vi "Text control 2 v6.5_pump-specific.vi"() -> ()   [LabVIEW 2016]
panel:
  in  "Tab Control":enum32{"Main", "Other parameters"}(tab)
  out "Line running":i32
  out "Total lines":i32
  out "Path":path=path "C:/users/rlp38/09Apr2009LTtesting/test2.txt"
  out "I vs Vg":cluster{"Y data in":dbl[], "X data in":dbl[]}[](graph)
  out "Is max":dbl format="%.2e"
  out "Id max":dbl format="%.2e"
  out "Ig max":dbl format="%.2e"
  out "Imax vs time":cluster{"Y data in":dbl[], "X data in":dbl[]}[](graph)
  out "Imin vs time":cluster{"Y data in":dbl[], "X data in":dbl[]}[](graph)
  out "I vs Vd":cluster{"Y data in":dbl[], "X data in":dbl[]}[](graph)
  in  "Script":string="#-------------------------------------------------------\n# SPM pump cleaning script\n#\n# Version: 0.5\n# Author: Dimitrios Simatos\n# Last updated: 2018-01-05\n#-------------------------------------------------------\n# Description\n#\n# This script is designed to run the cleaning sequence of the SPM OEM pump.\n# This script needs to be run 4 times!\n#-------------------------------------------------------\n# Changes\n#\n# Placed initialization and hard stop commands in the beginning.\n#-------------------------------------------------------\n# Important points\n#\n# Never leave any liquid in the pump to dry after the experiments. If they dry, the residue may block the valve.\n# Always run the cleaning cycle after the experiments.\n# Use clockwise rotation when going up in valve port numbers and vice versa.\n#-------------------------------------------------------\n# Things to do before running the script\n#\n# Set time units to minutes.\n# Set filenames.\n# Replace the tubing, if necessary.\n#-------------------------------------------------------\n# Port connections\n#\n# Port 1: Waste\n# Port 2: Waste\n# Port 3: Various cleaning liquids\n# Port 4: Waste\n# Port 5: Waste\n# Port 6: Waste\n#\n# Between each of the 4 runs, the settings of Port 3 will change, according to the cleaning protocol.\n# The settings for Port 3 are:\n# 1st run: 1% v/v solution of sodium hypochlorite in ultrapure water\n# 2nd run: 0.1% w/v solution of sodium dodecyl sulfate in ultrapure water\n# 3rd run: Ultrapure water\n# 4th run: Waste (in air, not immersed in liquid)\n#-------------------------------------------------------\n# Cleaning protocol for the SPM OEM pump (from the manual)\n#\n# A cleaning procedure should be performed at the end of each day or in between two different experiments.\n# An effective cleaning can be performed in the following manner:\n# • Bleach solution to kill microorganisms\n# 1. Prepare a solution of 1% chlorine bleach and deionized water\n#    NOTE: Prepare a 1% v/v solution of sodium hypochlorite in deionized water\n# 2. Prepare a reservoir and place 1 tubing in the bleach solution and 5 tubings in a waste recipient\n# 3. Pick up the bleach solution through 1 port to entirely fill the syringe\n# 4. Sequentially output the syringe content through the remaining ports and throw it to the waste\n# 5. Repeat operation at least 2 times\n# • Detergent solution to remove debris\n# 1. Prepare a solution of 0.1% detergent and deionized water\n#    NOTE: Prepare a 0.1% w/v solution of sodium dodecyl sulfate in deionized water\n# 2. Move the tubing from the bleach solution reservoir and place it into a reservoir of detergent solution\n# 3. Pick up the detergent solution through 1 port to entirely fill the syringe\n# 4. Sequentially output the detergent solution through the remaining ports into the waste recipient\n# 5. Repeat operation at least 2 times\n# • Rinsing water to prepare the pump for your next experiment\n# 1. Move the tubing from the detergent solution reservoir and place it into a reservoir of deionized water\n# 2. Pick up the rinsing solution through 1 port to entirely fill the syringe\n# 3. Sequentially output the rinse water through the remaining ports into the waste recipient\n# 4. Repeat operation at least 2 times\n# • Replace the tubing, if necessary\n#-------------------------------------------------------\n# Pumping cycles and execution time\n#\n# Execution time for a single cycle: 6 x (1 min + 10 sec) = 7 minutes\n# Total execution time: 4 x 7 = 28 minutes\n# Since the script has to run 4 times, the cleaning lasts for: 4 x 28 = 112 minutes\n# Air must be the last to be pumped through the valve, to remove all liquids.\n# There are 4 pumping cycles. Each one draws a different liquid through port 3 and pumps it sequentially through ports 1,2,4,5,6.\n# During the sequential pumping, each port receives 200 ml of liquid (20% of the total syringe volume = 600 \"plunger units\")\n# The device must be disconnected from the port during the cleaning procedure.\n# All cycles are similar, except cycle 1 has the initialization command uncommented and the first report valve command commented.\n#-------------------------------------------------------\n# Volume of liquid needed\n#\n# Volume of liquid needed per cycle: 1 ml\n# Total volume of liquid needed per script run: 4 x 1 = 4 ml\n# Since the script has to run 4 times, the first 3 with different liquids, I need:\n# 4 ml of 1% v/v solution of sodium hypochlorite in ultrapure water\n# 4 ml of 0.1% w/v solution of sodium dodecyl sulfate in ultrapure water\n# 4 ml of ultrapure water\n#-------------------------------------------------------\n# Parameters\n#\n# Syringe size: 1 ml\n# Step resolution N = 0.01 mm\n# Drawing flow V = 300 pulses/second (6000 ul/min)\n# Pumping flow V = 300 pulses/second (6000 ul/min)\n#-------------------------------------------------------\n# Pump initialization\npump /1T #hard stop pump\npump /1ZR #initialize pump\n#-------------------------------------------------------\n# Cycle 1\n# Fill the syringe\npump /1Q #query pump\npump /1? #report absolute plunger position\n#pump /1?6 #report valve position\nwait-min 1 #wait 1 minute\npump /1N0R #set step resolution: 0.01 mm\npump /1Q #query pump\npump /1? #report absolute plunger position (the plunger should be at 0)\npump /1?6 #report valve position\nwait 1000 #wait 1 second\npump /1V300R #choose speed: 300 steps/s (6000 ul/min)\npump /1Q #query pump\nwait 1000 #wait 1 second\npump /1I3R #go to port 3, clockwise rotation\npump /1Q #query pump\npump /1?6 #report valve position\nwait 1000 #wait 1 second\npump /1A3000R #go to absolute position 3000 (= draw 1 ml)\nwait 30000 #wait 30 seconds\npump /1Q #query pump\npump /1? #report absolute plunger position (the plunger should have finished moving)\n#pump /1?6 #report valve position\n# The sequential pumping begins\n# Port 1\npump /1O1R #switch to port 1, counterclockwise rotation\npump /1Q #query pump\npump /1?6 #report valve position\npump /1A2400R #go to absolute position 2400 (= pump 200 ul)\npump /1Q #query pump\npump /1? #report absolute plunger position (the plunger should be moving to 0)\nwait-min 1 #wait 1 minute\npump /1? #report absolute plunger position (the plunger should have finished moving)\n# Port 2\npump /1I2R #switch to port 2, clockwise rotation\npump /1Q #query pump\npump /1?6 #report valve position\npump /1A1800R #go to absolute position 1800 (= pump 200 ul)\npump /1Q #query pump\npump /1? #report absolute plunger position (the plunger should be moving to 0)\nwait-min 1 #wait 1 minute\npump /1? #report absolute plunger position (the plunger should have finished moving)\n# Port 4\npump /1I4R #switch to port 4, clockwise rotation\npump /1Q #query pump\npump /1?6 #report valve position\npump /1A1200R #go to absolute position 1200 (= pump 200 ul)\npump /1Q #query pump\npump /1? #report absolute plunger position (the plunger should be moving to 0)\nwait-min 1 #wait 1 minute\npump /1? #report absolute plunger position (the plunger should have finished moving)\n# Port 5\npump /1I5R #switch to port 5, clockwise rotation\npump /1Q #query pump\npump /1?6 #report valve position\npump /1A600R #go to absolute position 600 (= pump 200 ul)\npump /1Q #query pump\npump /1? #report absolute plunger position (the plunger should be moving to 0)\nwait-min 1 #wait 1 minute\npump /1? #report absolute plunger position (the plunger should have finished moving)\n# Port 6\npump /1I6R #switch to port 6, clockwise rotation\npump /1Q #query pump\npump /1?6 #report valve position\npump /1A0R #go to absolute position 0 (= pump 200 ul)\npump /1Q #query pump\npump /1? #report absolute plunger position (the plunger should be moving to 0)\nwait-min 1 #wait 1 minute\npump /1? #report absolute plunger position (the plunger should have finished moving)\n#-------------------------------------------------------\n# Cycle 2\n# Fill the syringe\n#pump /1ZR #initialize pump\npump /1Q #query pump\npump /1? #report absolute plunger position\npump /1?6 #report valve position\nwait-min 1 #wait 1 minute\npump /1N0R #set step resolution: 0.01 mm\npump /1Q #query pump\npump /1? #report absolute plunger position (the plunger should be at 0)\npump /1?6 #report valve position\nwait 1000 #wait 1 second\npump /1V300R #choose speed: 300 steps/s (6000 ul/min)\npump /1Q #query pump\nwait 1000 #wait 1 second\npump /1O3R #go to port 3, counterclockwise rotation\npump /1Q #query pump\npump /1?6 #report valve position\nwait 1000 #wait 1 second\npump /1A3000R #go to absolute position 3000 (= draw 1 ml)\nwait 30000 #wait 30 seconds\npump /1Q #query pump\npump /1? #report absolute plunger position (the plunger should have finished moving)\n#pump /1?6 #report valve position\n# The sequential pumping begins\n# Port 1\npump /1O1R #switch to port 1, counterclockwise rotation\npump /1Q #query pump\npump /1?6 #report valve position\npump /1A2400R #go to absolute position 2400 (= pump 200 ul)\npump /1Q #query pump\npump /1? #report absolute plunger position (the plunger should be moving to 0)\nwait-min 1 #wait 1 minute\npump /1? #report absolute plunger position (the plunger should have finished moving)\n# Port 2\npump /1I2R #switch to port 2, clockwise rotation\npump /1Q #query pump\npump /1?6 #report valve position\npump /1A1800R #go to absolute position 1800 (= pump 200 ul)\npump /1Q #query pump\npump /1? #report absolute plunger position (the plunger should be moving to 0)\nwait-min 1 #wait 1 minute\npump /1? #report absolute plunger position (the plunger should have finished moving)\n# Port 4\npump /1I4R #switch to port 4, clockwise rotation\npump /1Q #query pump\npump /1?6 #report valve position\npump /1A1200R #go to absolute position 1200 (= pump 200 ul)\npump /1Q #query pump\npump /1? #report absolute plunger position (the plunger should be moving to 0)\nwait-min 1 #wait 1 minute\npump /1? #report absolute plunger position (the plunger should have finished moving)\n# Port 5\npump /1I5R #switch to port 5, clockwise rotation\npump /1Q #query pump\npump /1?6 #report valve position\npump /1A600R #go to absolute position 600 (= pump 200 ul)\npump /1Q #query pump\npump /1? #report absolute plunger position (the plunger should be moving to 0)\nwait-min 1 #wait 1 minute\npump /1? #report absolute plunger position (the plunger should have finished moving)\n# Port 6\npump /1I6R #switch to port 6, clockwise rotation\npump /1Q #query pump\npump /1?6 #report valve position\npump /1A0R #go to absolute position 0 (= pump 200 ul)\npump /1Q #query pump\npump /1? #report absolute plunger position (the plunger should be moving to 0)\nwait-min 1 #wait 1 minute\npump /1? #report absolute plunger position (the plunger should have finished moving)\n#-------------------------------------------------------\n# Cycle 3\n# Fill the syringe\n#pump /1ZR #initialize pump\npump /1Q #query pump\npump /1? #report absolute plunger position\npump /1?6 #report valve position\nwait-min 1 #wait 1 minute\npump /1N0R #set step resolution: 0.01 mm\npump /1Q #query pump\npump /1? #report absolute plunger position (the plunger should be at 0)\npump /1?6 #report valve position\nwait 1000 #wait 1 second\npump /1V300R #choose speed: 300 steps/s (6000 ul/min)\npump /1Q #query pump\nwait 1000 #wait 1 second\npump /1O3R #go to port 3, counterclockwise rotation\npump /1Q #query pump\npump /1?6 #report valve position\nwait 1000 #wait 1 second\npump /1A3000R #go to absolute position 3000 (= draw 1 ml)\nwait 30000 #wait 30 seconds\npump /1Q #query pump\npump /1? #report absolute plunger position (the plunger should have finished moving)\n#pump /1?6 #report valve position\n# The sequential pumping begins\n# Port 1\npump /1O1R #switch to port 1, counterclockwise rotation\npump /1Q #query pump\npump /1?6 #report valve position\npump /1A2400R #go to absolute position 2400 (= pump 200 ul)\npump /1Q #query pump\npump /1? #report absolute plunger position (the plunger should be moving to 0)\nwait-min 1 #wait 1 minute\npump /1? #report absolute plunger position (the plunger should have finished moving)\n# Port 2\npump /1I2R #switch to port 2, clockwise rotation\npump /1Q #query pump\npump /1?6 #report valve position\npump /1A1800R #go to absolute position 1800 (= pump 200 ul)\npump /1Q #query pump\npump /1? #report absolute plunger position (the plunger should be moving to 0)\nwait-min 1 #wait 1 minute\npump /1? #report absolute plunger position (the plunger should have finished moving)\n# Port 4\npump /1I4R #switch to port 4, clockwise rotation\npump /1Q #query pump\npump /1?6 #report valve position\npump /1A1200R #go to absolute position 1200 (= pump 200 ul)\npump /1Q #query pump\npump /1? #report absolute plunger position (the plunger should be moving to 0)\nwait-min 1 #wait 1 minute\npump /1? #report absolute plunger position (the plunger should have finished moving)\n# Port 5\npump /1I5R #switch to port 5, clockwise rotation\npump /1Q #query pump\npump /1?6 #report valve position\npump /1A600R #go to absolute position 600 (= pump 200 ul)\npump /1Q #query pump\npump /1? #report absolute plunger position (the plunger should be moving to 0)\nwait-min 1 #wait 1 minute\npump /1? #report absolute plunger position (the plunger should have finished moving)\n# Port 6\npump /1I6R #switch to port 6, clockwise rotation\npump /1Q #query pump\npump /1?6 #report valve position\npump /1A0R #go to absolute position 0 (= pump 200 ul)\npump /1Q #query pump\npump /1? #report absolute plunger position (the plunger should be moving to 0)\nwait-min 1 #wait 1 minute\npump /1? #report absolute plunger position (the plunger should have finished moving)\n#-------------------------------------------------------\n# Cycle 4\n# Fill the syringe\n#pump /1ZR #initialize pump\npump /1Q #query pump\npump /1? #report absolute plunger position\npump /1?6 #report valve position\nwait-min 1 #wait 1 minute\npump /1N0R #set step resolution: 0.01 mm\npump /1Q #query pump\npump /1? #report absolute plunger position (the plunger should be at 0)\npump /1?6 #report valve position\nwait 1000 #wait 1 second\npump /1V300R #choose speed: 300 steps/s (6000 ul/min)\npump /1Q #query pump\nwait 1000 #wait 1 second\npump /1O3R #go to port 3, counterclockwise rotation\npump /1Q #query pump\npump /1?6 #report valve position\nwait 1000 #wait 1 second\npump /1A3000R #go to absolute position 3000 (= draw 1 ml)\nwait 30000 #wait 30 seconds\npump /1Q #query pump\npump /1? #report absolute plunger position (the plunger should have finished moving)\n#pump /1?6 #report valve position\n# The sequential pumping begins\n# Port 1\npump /1O1R #switch to port 1, counterclockwise rotation\npump /1Q #query pump\npump /1?6 #report valve position\npump /1A2400R #go to absolute position 2400 (= pump 200 ul)\npump /1Q #query pump\npump /1? #report absolute plunger position (the plunger should be moving to 0)\nwait-min 1 #wait 1 minute\npump /1? #report absolute plunger position (the plunger should have finished moving)\n# Port 2\npump /1I2R #switch to port 2, clockwise rotation\npump /1Q #query pump\npump /1?6 #report valve position\npump /1A1800R #go to absolute position 1800 (= pump 200 ul)\npump /1Q #query pump\npump /1? #report absolute plunger position (the plunger should be moving to 0)\nwait-min 1 #wait 1 minute\npump /1? #report absolute plunger position (the plunger should have finished moving)\n# Port 4\npump /1I4R #switch to port 4, clockwise rotation\npump /1Q #query pump\npump /1?6 #report valve position\npump /1A1200R #go to absolute position 1200 (= pump 200 ul)\npump /1Q #query pump\npump /1? #report absolute plunger position (the plunger should be moving to 0)\nwait-min 1 #wait 1 minute\npump /1? #report absolute plunger position (the plunger should have finished moving)\n# Port 5\npump /1I5R #switch to port 5, clockwise rotation\npump /1Q #query pump\npump /1?6 #report valve position\npump /1A600R #go to absolute position 600 (= pump 200 ul)\npump /1Q #query pump\npump /1? #report absolute plunger position (the plunger should be moving to 0)\nwait-min 1 #wait 1 minute\npump /1? #report absolute plunger position (the plunger should have finished moving)\n# Port 6\npump /1I6R #switch to port 6, clockwise rotation\npump /1Q #query pump\npump /1?6 #report valve position\npump /1A0R #go to absolute position 0 (= pump 200 ul)\npump /1Q #query pump\npump /1? #report absolute plunger position (the plunger should be moving to 0)\nwait-min 1 #wait 1 minute\npump /1? #report absolute plunger position (the plunger should have finished moving)\n#-------------------------------------------------------"
  out "Command running:":string
  out "Serial port data":string
  out "Elapsed Time":dbl caption="Elapsed Time (s)"
  in  "Time Units":u16(ring)=1 items=["Seconds", "Minutes", "Hours"]
  in  "Time Offset":dbl caption="Set Start Time (s)"
  in  "Reset":bool
  in  "Auto Reset":bool
  in  "integration time":u32(slide) max=2 step=1 scale=0.0..2.0
  in  "Interrupt scan":bool
  out "Absolute plunger position vs time":cluster{"Y data in":dbl[], "X data in":dbl[]}[](graph)
  out "Valve position vs time":cluster{"Y data in":dbl[], "X data in":dbl[]}[](graph)
  out "Is on":dbl format="%.2e"
  out "Id on":dbl format="%.2e"
  out "Ig on":dbl format="%.2e"
  out "Ion vs time":cluster{"Y data in":dbl[], "X data in":dbl[]}[](graph)
  out "Ioff vs time":cluster{"Y data in":dbl[], "X data in":dbl[]}[](graph)
  out "Ig min":dbl format="%.2e"
  out "Id min":dbl format="%.2e"
  out "Is min":dbl format="%.2e"
  out "Is off":dbl format="%.2e"
  out "Id off":dbl format="%.2e"
  out "Ig off":dbl format="%.2e"
  in  "Integration time (long)":dbl=0.32 min=0.04 max=2.0 step=0.02 format="%.2f"
  in  "Integration time (short)":dbl=0.0019 min=8e-05 max=0.0019 step=8e-05 format="%^.0e"
  in  "Gate: Compliance":dbl=0.001 format="%.8f"
  in  "Drain: Compliance":dbl=0.001 format="%.8f"
  in  "Hard stop pump":bool
  in  "Halt pump":bool
  in  "Interrupt program":bool
  in  "Suffix (script)":string="step_1_up-H2O_initial_script.txt"
  in  "Filename (variable part)":string="step_1_up-H2O_initial_"
  in  "Plot output curve extrema vs time":bool
  in  "Plot transfer curve extrema vs time":bool=TRUE
  in  "Gate Range\nmode":u16(ring) items=["Auto", "Limited", "Fixed"]
  in  "Gate Range":u8(slide)=6 max=11 scale=0.0..11.0
  in  "Source/Drain\nRange mode":u16(ring) items=["Auto", "Limited", "Fixed"]
  in  "Source/Drain Range":u8(slide)=6 max=11 scale=0.0..11.0
  in  "Panel Controls":T1={"Emergency Stop"=refnum, "TransGraph Max"=1e-05, "Text/Graph (text=false)"=TRUE} {"TransGraph Max" format="%.2e"}
  in  "Panel Controls 2":T2={"Emergency Stop"=refnum, "TransGraph Max"=1e-05, "Text/Graph (text=false)"=TRUE, "TransGraph Min"=1e-11} {"TransGraph Min" format="%.2e"; "TransGraph Max" format="%.2e"}
  in  "SMU4":cluster{"on/off":bool, "Voltage":dbl} {"Voltage" min=-100.0 max=100.0 format="%.2f"}
  in  "Full Reset":bool
  in  "Standby":T3
  out "error out":errorcluster
  in  "Delay before read (ms)":u32=1000
  in  "byte count":u32=64
  in  "Serial End Mode for Reads":u16(ring)=2 items=["None", "LastBit", "TermChar"]
  in  "Timeout (ms)":u32=10000
  in  "Enable Termination\nChar (T)":bool=TRUE
  in  "Termination char\n(0xA = '\\n' = LF)\n(0xD = '\\r' = CR)":u8=13 format="%.0x"
  in  "flow control":u16(ring) items=["None"=0, "XON/XOFF"=1, "RTS/CTS"=2, "DTR/DSR"=4]
  in  "stop bits":u16(ring)=10 items=["1.0"=10, "1.5"=15, "2.0"=20]
  in  "parity":u16(ring) items=["None", "Odd", "Even", "Mark", "Space"]
  in  "data bits":u16=8 min=5 max=8 step=1
  in  "VISA resource name":refnum<visa-resource-name>="COM6"
  in  "baud rate":u32=9600
  out "Timings Indicator":T4
  in  "Timings (overwritten by the Front Panel)":T5={"integration time"=0, "Short/Long integration time"=0.00064, "hold time (sec)"=0.0, "delay time (sec)"=0.0, "Step Time (0 disables)"=0.0, "sweep method"=0, "Pulse period"=0.005, "Base voltage"=0.0, "Pulse width"=0.0005} {"Pulse width" min=0.0005 max=0.1 step=0.0001 format="%.4f"; "Base voltage" format="%^.4e"; "Pulse period" min=0.005 max=1.0 step=0.0001 format="%.4f"; "sweep method" items=["Continuous", "Pulsed"]; "Step Time (0 disables)" format="%.2f"; "delay time (sec)" format="%.4f"; "hold time (sec)" format="%.4f"; "Short/Long integration time" format="%^.0e"; "integration time" scale=0.0..2.0}
  out "SMU4 Indicator":cluster{"on/off":bool, "Voltage":dbl} {"Voltage" min=-100.0 max=100.0 format="%.2f"}
  in  "Gate":T6={"Gate Start"=0.0, "Gate Stop"=2.0, "Gate Step (linear only)"=1.0, "Gate Compliance"=0.0001, "Gate PComp"=0.0, "Range mode"=0, "Range"=6} {"Range" max=11 scale=0.0..11.0; "Range mode" items=["Auto", "Limited", "Fixed"]; "Gate PComp" format="%^.2e"; "Gate Compliance" format="%^.2e"; "Gate Step (linear only)" format="%^.4e"; "Gate Stop" format="%^.4e"; "Gate Start" format="%^.4e"}
  in  "Drain 2":T7={"Drain Start"=0.0, "Drain Stop"=2.0, "Drain Compliance"=0.0001, "Drain Step"=1.0, "Drain PComp"=0.0, "Range mode"=0, "Range"=6} {"Range" max=11 scale=0.0..11.0; "Range mode" items=["Auto", "Limited", "Fixed"]; "Drain PComp" format="%^.2e"; "Drain Step" format="%^.4e"; "Drain Compliance" format="%^.2e"; "Drain Stop" format="%^.4e"; "Drain Start" format="%^.4e"}
  # "Syntax:\nitime [s|m|l] time(sec): [s|m|l] determines the integration time setting (small|medium|long) and time sets the value.\nNOTE: The value of the integration time has to be within the range allowed by its category (s|m|l), otherwise, the closest value will be used. (e.g. if the category is set to short but the time value is very long, the actual value used will be the maximum short integration time.\nIntegration times:\n    Short: Default: 640 us. Range: 8E-5 - 1.92E-3 seconds.\n    Medium: Fixed at 1 NPL cycle (0.02 seconds).\n    Long: Default: 16 NPL cycles (0.32 seconds). Range: 2-100 NPL cycles (0.04 seconds - 2 seconds).\ngaterangemode [a|l|f]\ndrainrangemode [a|l|f]\npulsed [on|off] PulsePeriod(sec) PulseBaseVoltage PulseONWidth(sec)\nstandby [on l off]\nwait NumMilliseconds\nwait-min NumMinutes\n# texthere = comment\nSMU4 [ON|OFF] Voltage\ntransfer [s|d] VgStart VgStop VgStep VdStart VdStop VdStep\noutput [s|d] VgStart VgStop VgStep VdStart VdStop VdStep\nsample Vg Vd NumSamples Time(s) SampleInterval(s)\nsamplei Idg NumSamples Time(s) SampleInterval(s) VDGcompliance\n100 samples is approximately 13 seconds with medium integration\n# if in doubt use SampleInterval(s) = 0.004\nstressV VG VD IGcompliance IDcompliance Duration(sec)\nstressI IDG VDGcompliance Duration(sec)\nvsu2pulse Bias Duration(s)\npulsedstressV [s|d] VEstop VgON VgOFF Period(s) PulseONwidth(s) Vd\nsample-fpp Vg Vd NumSamples Time\nresample-fpp Vg Vd\ntransfer-fpp [s|d] VgStart VgStop VgStep VdStart VdStop VdStep\noutput-fpp [s|d] VgStart VgStop VgStep VdStart VdStop VdStep\nserial SerialPortCommand\npump SerialPortCommand for the SPM pump\n\nSPM Pump Syntax (<x>: pump number, use 1 if only one pump):\nif the command syntax contains [R], then append the letter R to the command\n/<x>Q: query (a query command should follow each command)\n/<x>Z[R] or /<x>Y[R]: initialize pump\n/<x>N<n>[R] (<n>=0,1): <0> (<1>) microstep 0.01 mm (0.00125 mm) resolution\n/<x>I<n> (<n>=0-6): turn to port number n (clockwise)\n/<x>O<n> (<n>=0-6): turn to port number n (counterclockwise)\n/<x>X: Re-execute last command string\n/<x>G<n>[R] (<n>=0-60000): repeat command sequence (default: 0, 0=loop forever)\n/<x>g: Mark the start of a repeat sequence (max = 10)\n/<x>M<n>[R] (<n>=0-86400000): delay command execution by n milliseconds\n/<x>H: Halt; Pause the sequence after finishing the current move\n/<x>T: Hardstop; Interrupt the current move and suppress it from the sequence\n/<x>A<n>[R] (<n>=0-3000 with N=0, 0-24000 with N=1): absolute position\n/<x>P<n>[R] (<n>=0-3000 with N=0, 0-24000 with N=1): relative pickup\n/<x>D<n>[R] (<n>=0-3000 with N=0, 0-24000 with N=1): relative dispense\n/<x>V<n>[R] (<n>=1-1600 default: 150): set peak speed (pulses/sec)\nNOTE: The lowest speed limit is 1 pulse/sec, not 5, as the manual states.\n/<x>S<n>[R] (<n>=10-40 default: 22): set speed (NOT in pulses/sec, look in manual)\nNOTE: When controlled with absolute position, one does not need to pay special attention to the syringe that is mounted on the pump.\nWithdraw from lower stage (ports 3, 5), dispense from higher stage (ports 2, 4, 6).\nConnect Port 1 to waste."
  # "Time"
  # "1\n2\n3\n4\n5\n6\n7\n8\n9\n10\n11\n12\n13\n14\n15\n16\n17\n18\n19\n20"
  # "Serial port settings"
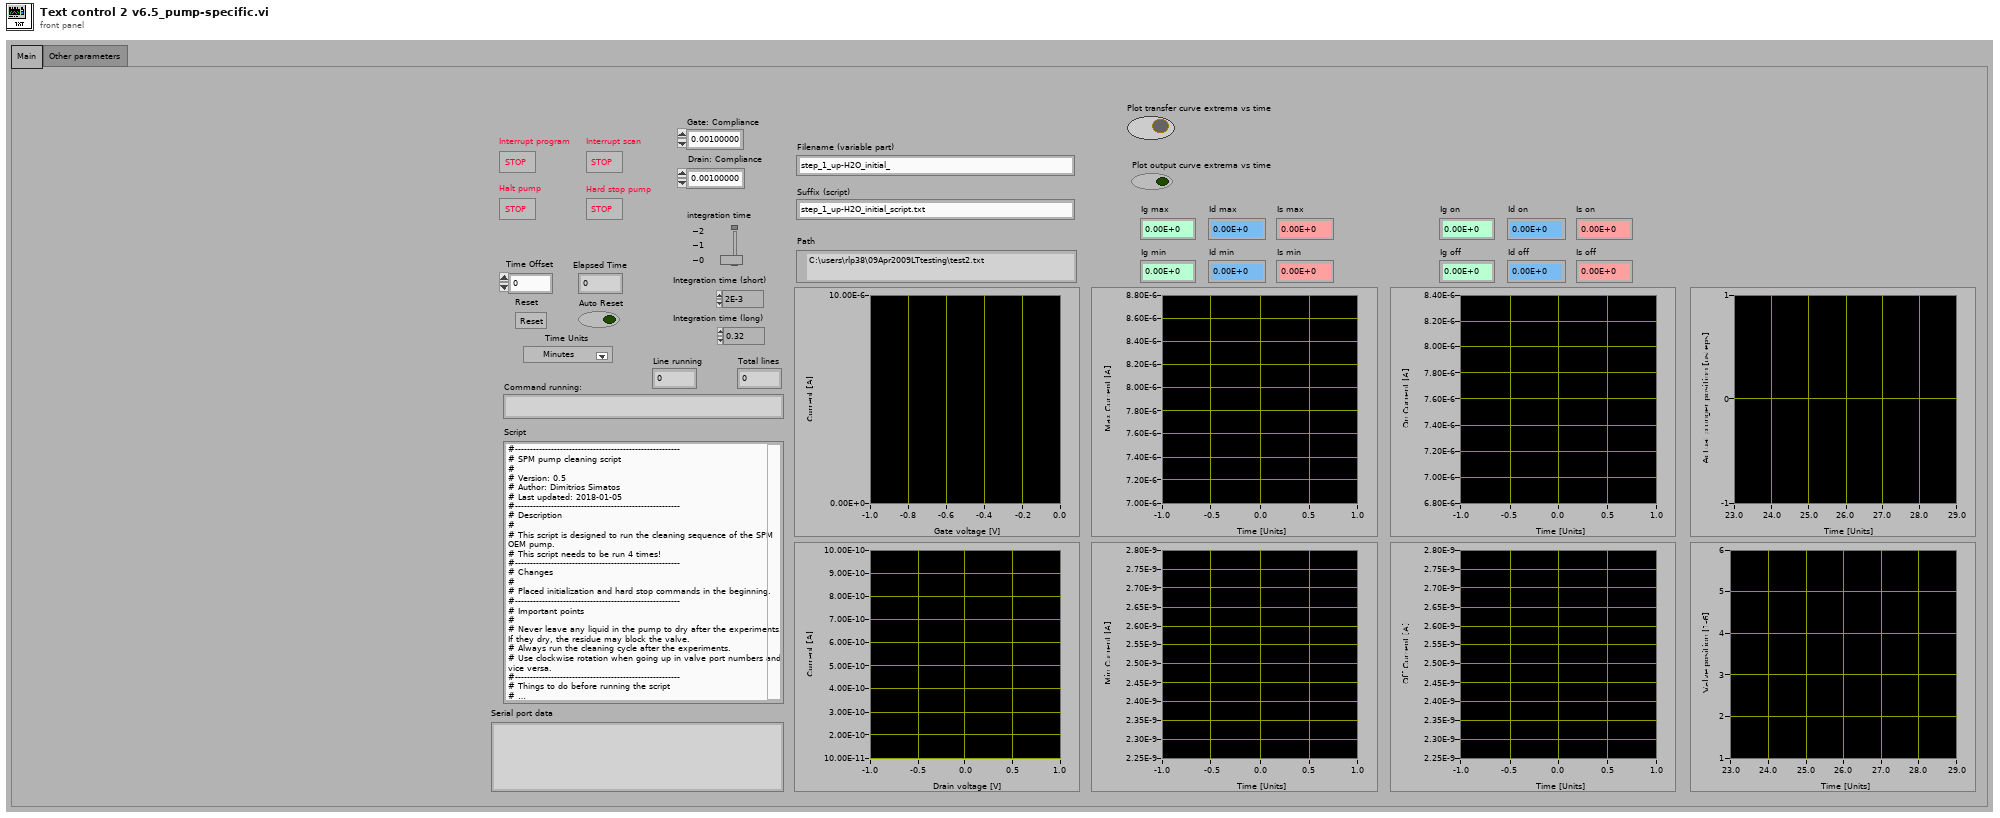
[diagram p1: front panel]
types:
  T1 = cluster{"Emergency Stop":refnum<vi>, "TransGraph Max":dbl, "Text/Graph (text=false)":bool}
  T2 = cluster{"Emergency Stop":refnum<vi>, "TransGraph Max":dbl, "Text/Graph (text=false)":bool, "TransGraph Min":dbl}
  T3 = cluster{"Gate Standby":bool, "Drain Standby":bool}
  T4 = cluster{"integration time (0:s, 1:m, 2:l)":u32, "Short/Long integration time":dbl, "hold time (sec)":dbl, "delay time (sec)":dbl, "Step Time (0 disables)":dbl, "sweep method":u16, "Pulse period":dbl, "Base voltage":dbl, "Pulse width":dbl}
  T5 = cluster{"integration time":u32, "Short/Long integration time":dbl, "hold time (sec)":dbl, "delay time (sec)":dbl, "Step Time (0 disables)":dbl, "sweep method":u16, "Pulse period":dbl, "Base voltage":dbl, "Pulse width":dbl}
  T6 = cluster{"Gate Start":dbl, "Gate Stop":dbl, "Gate Step (linear only)":dbl, "Gate Compliance":dbl, "Gate PComp":dbl, "Range mode":u16, "Range":u8}
  T7 = cluster{"Drain Start":dbl, "Drain Stop":dbl, "Drain Compliance":dbl, "Drain Step":dbl, "Drain PComp":dbl, "Range mode":u16, "Range":u8}
  T8 = enum16{"open", "replace", "create", "open or create", "replace or create", "replace or create with confirmation"}
  T9 = cluster{"V2 Start":dbl, "V2 Step":dbl, "Number of points":i32}
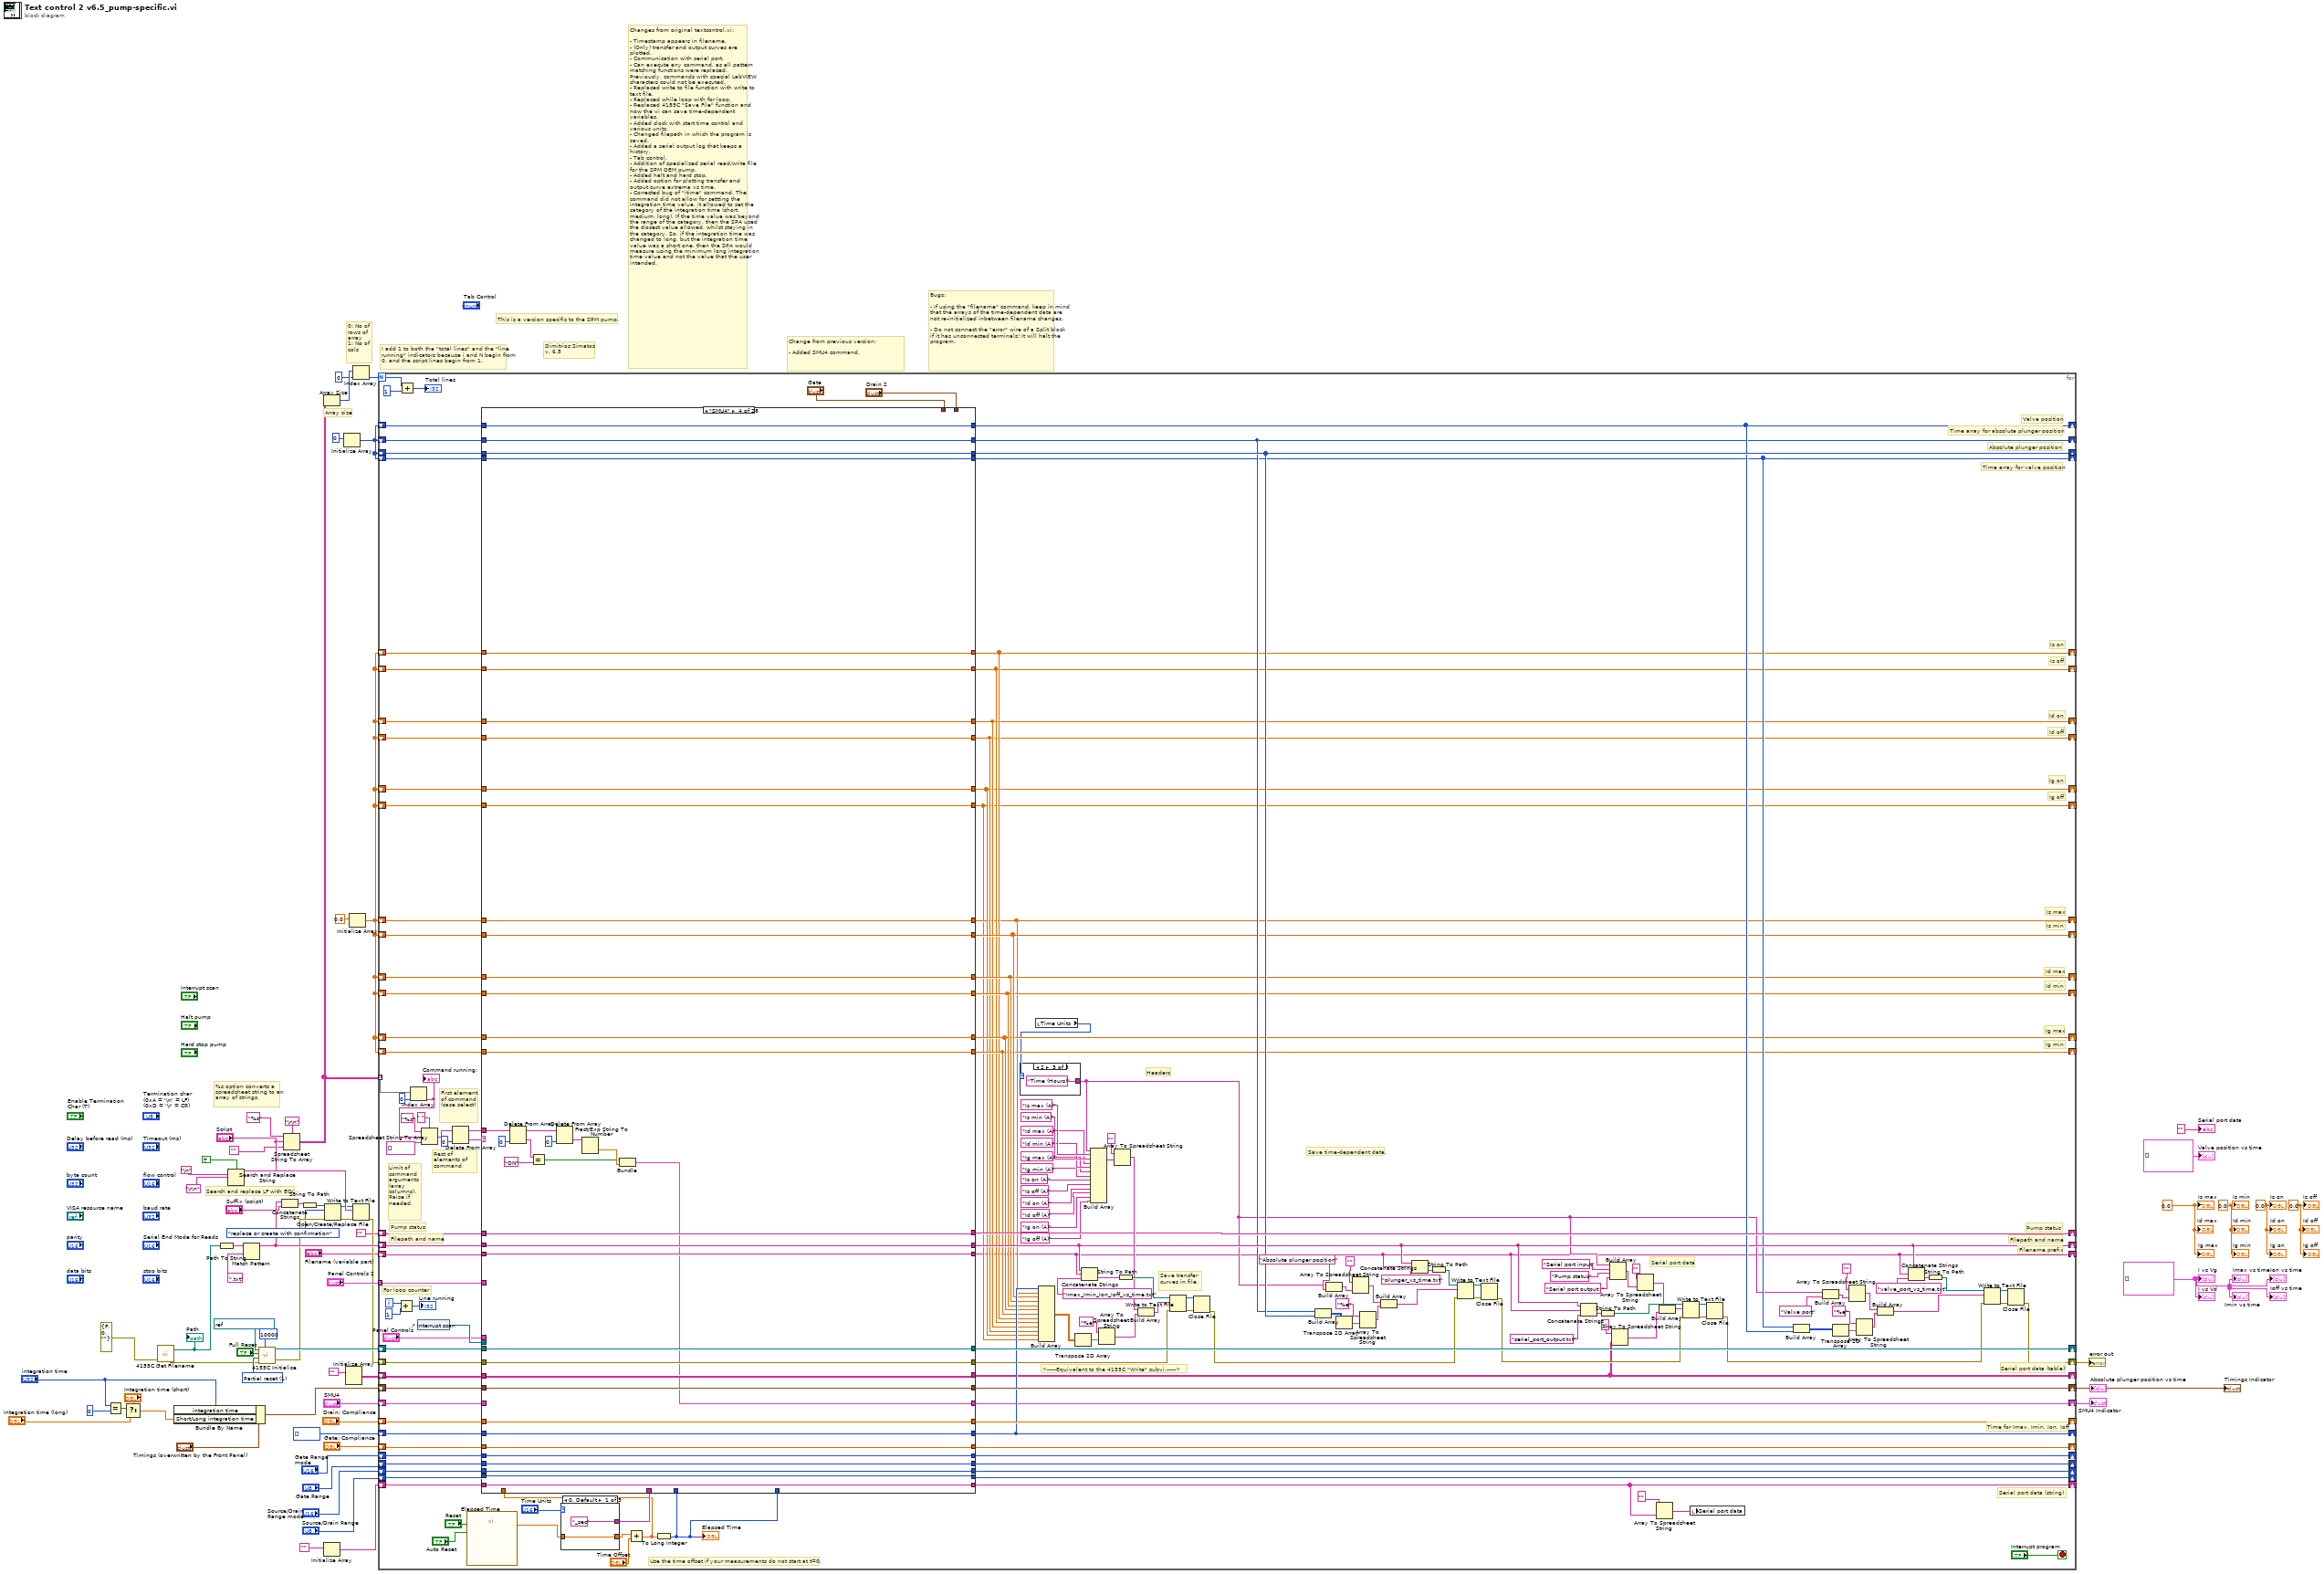
[diagram p0: block diagram]
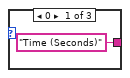
[diagram p2: hidden frame]
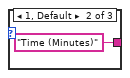
[diagram p3: hidden frame]
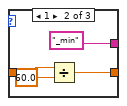
[diagram p4: hidden frame]
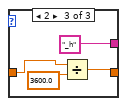
[diagram p5: hidden frame]
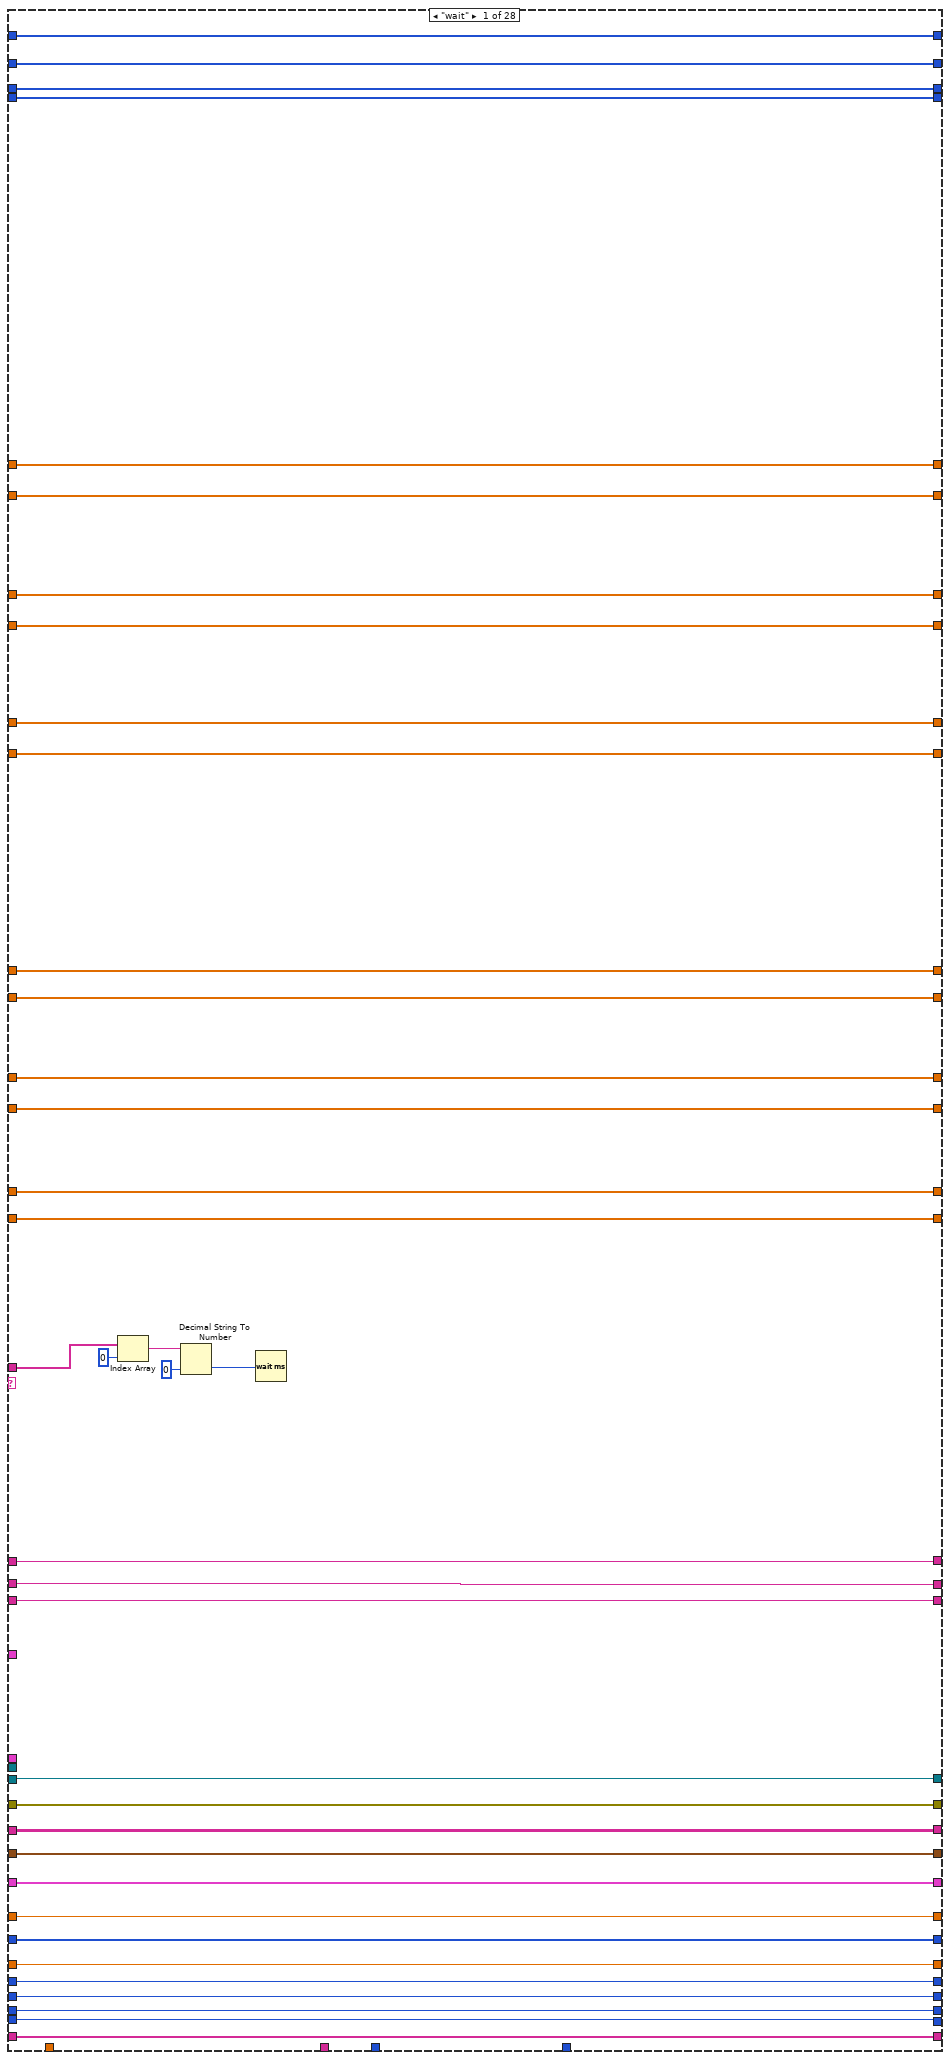
[diagram p6: hidden frame]
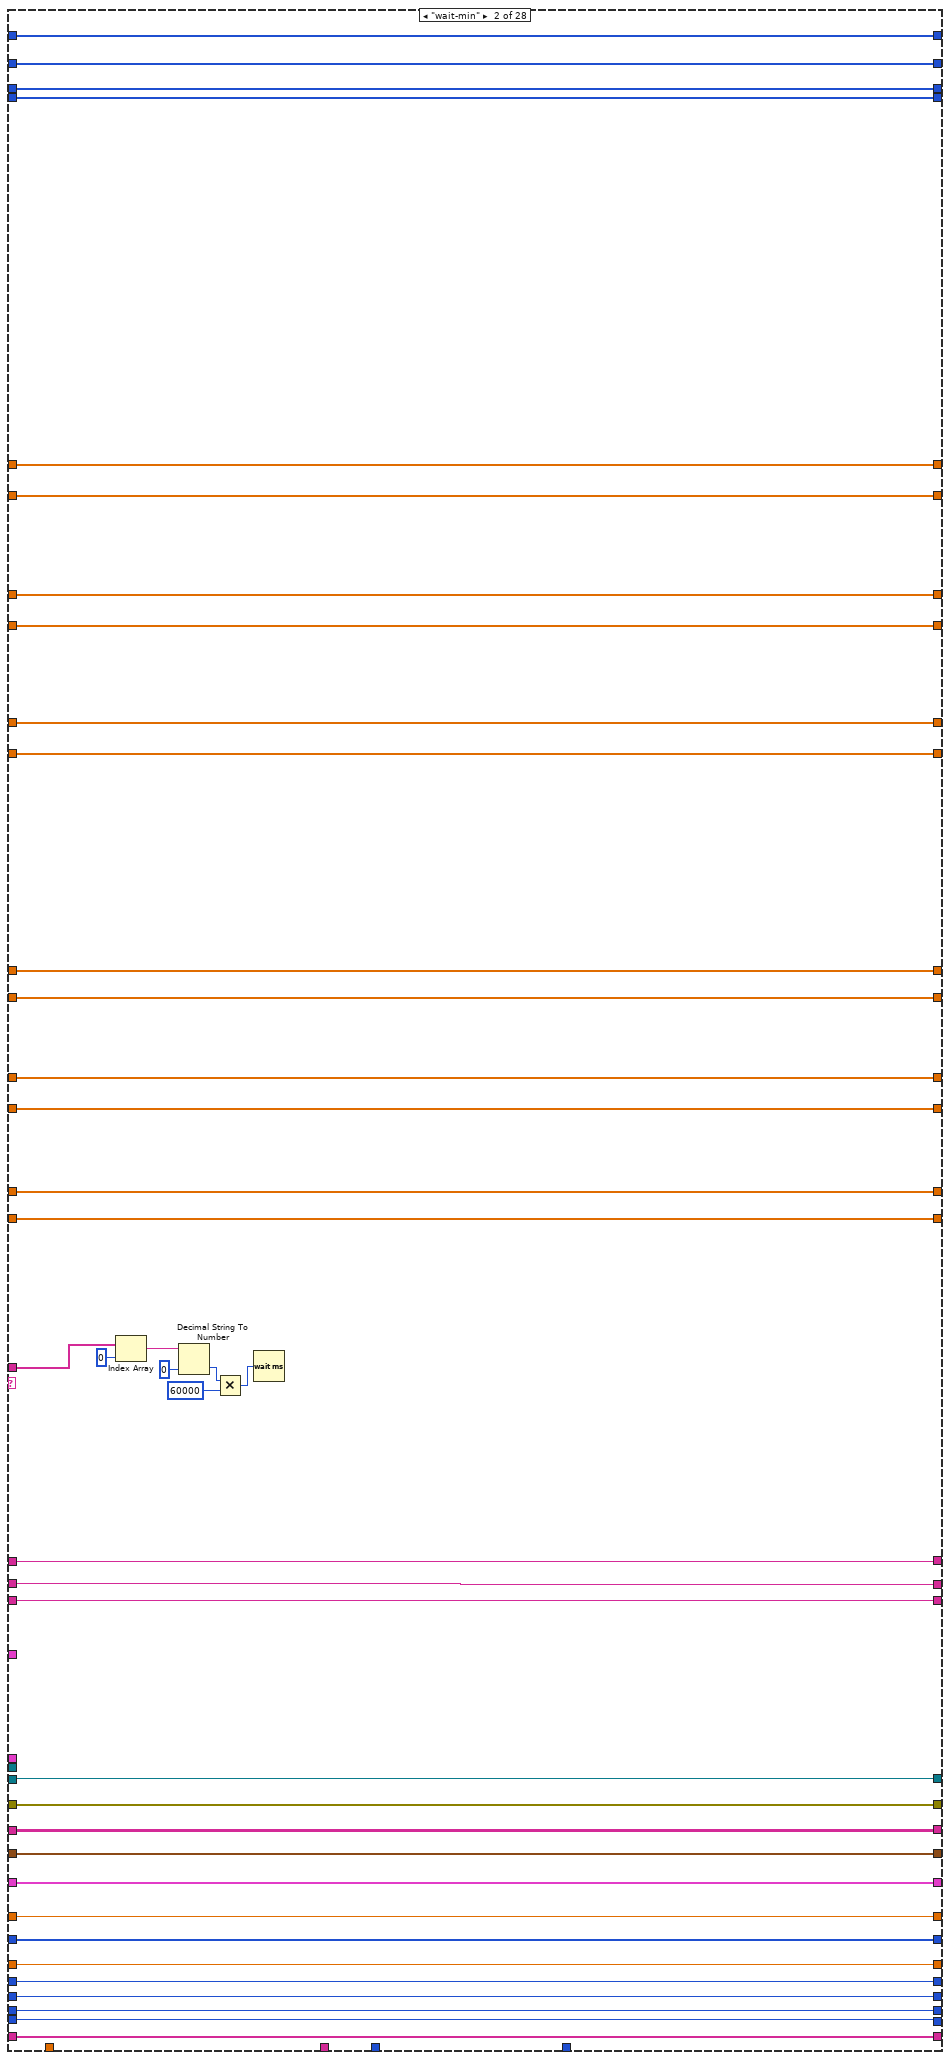
[diagram p7: hidden frame]
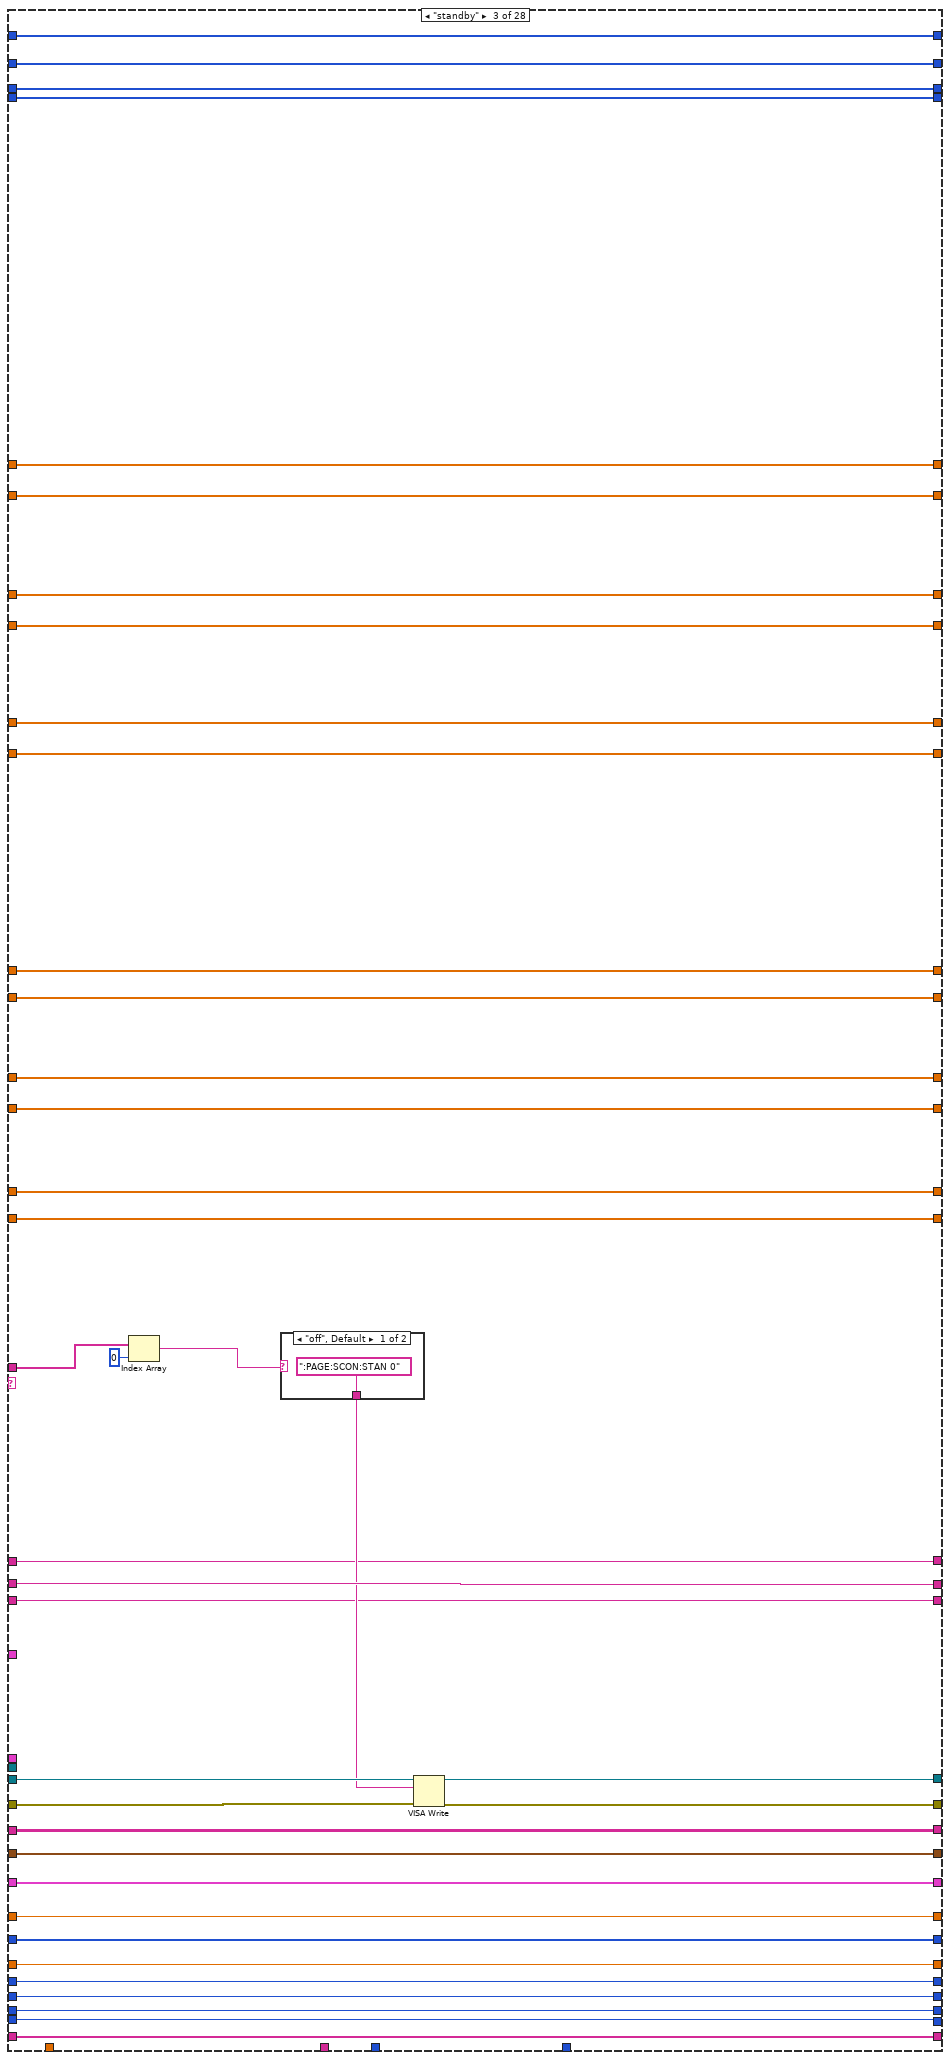
[diagram p8: hidden frame]
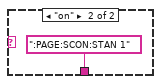
[diagram p9: hidden frame]
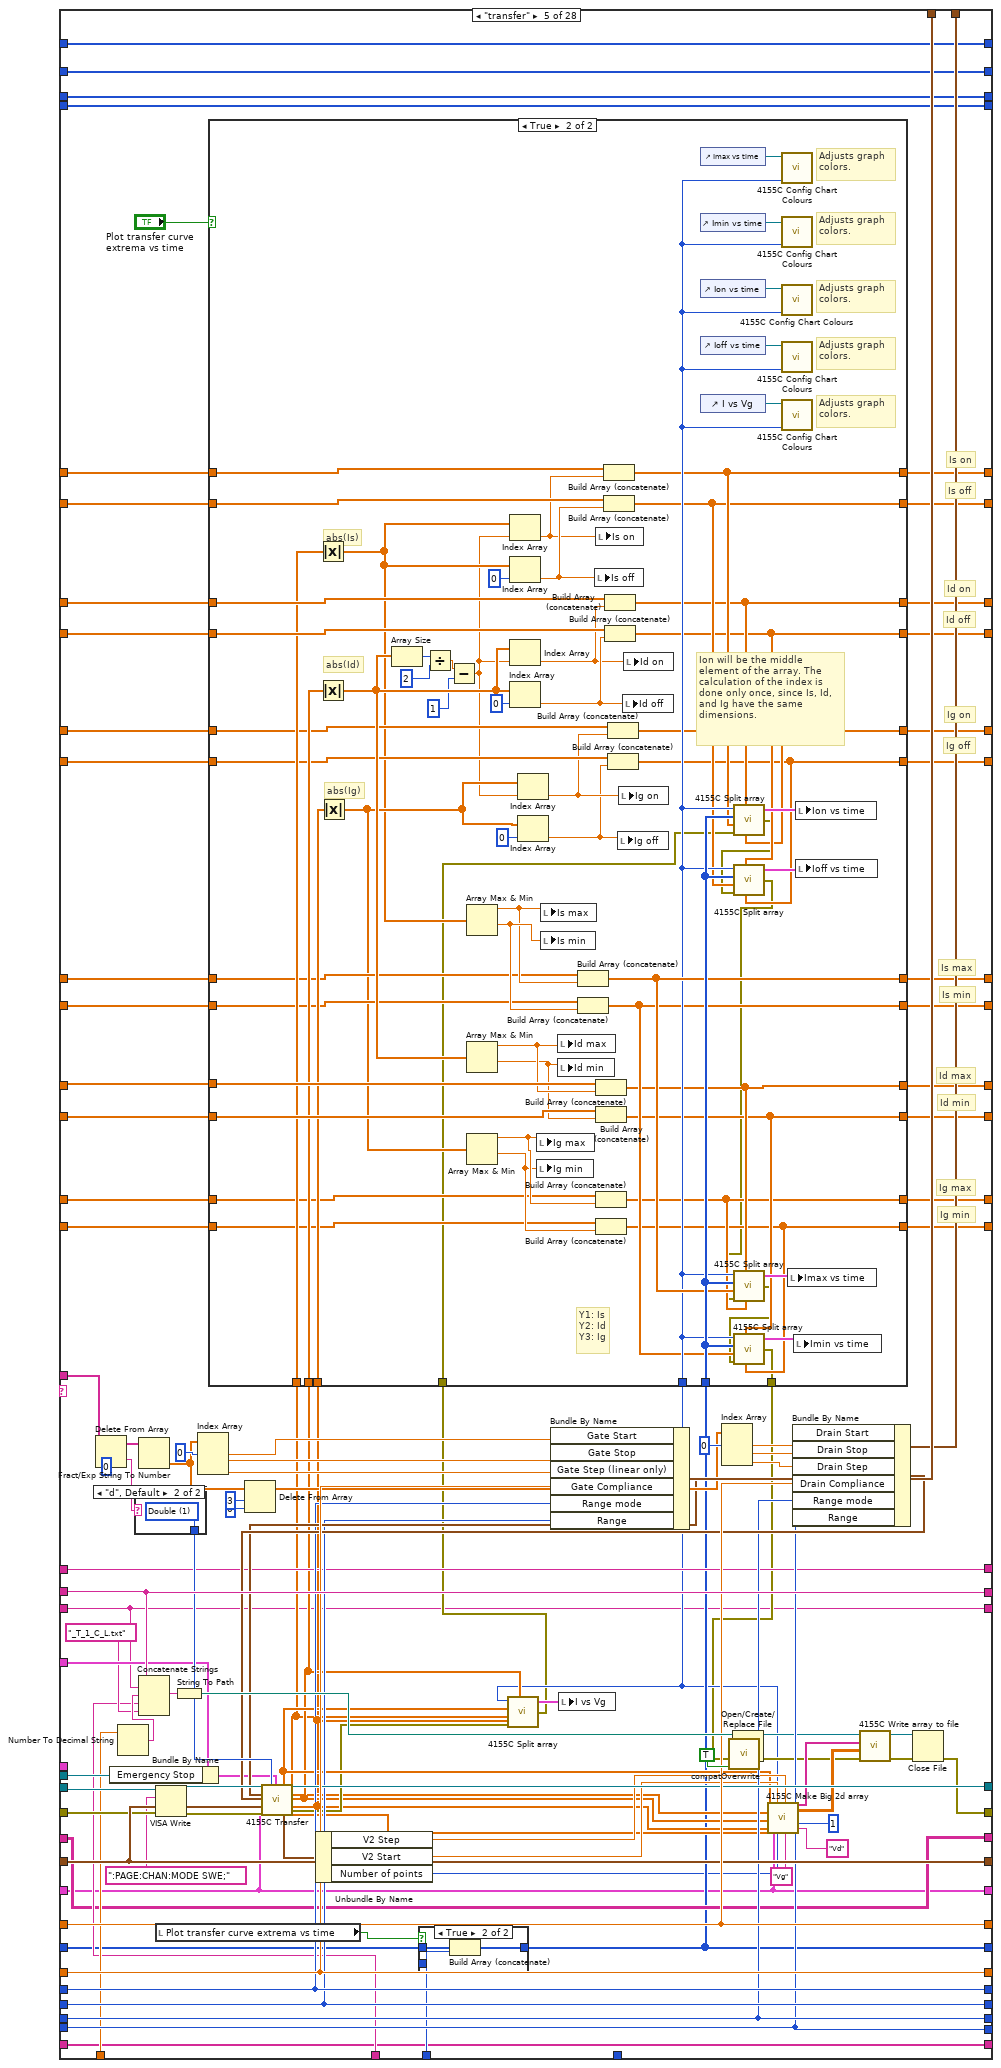
[diagram p10: hidden frame]
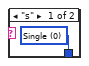
[diagram p13: hidden frame]
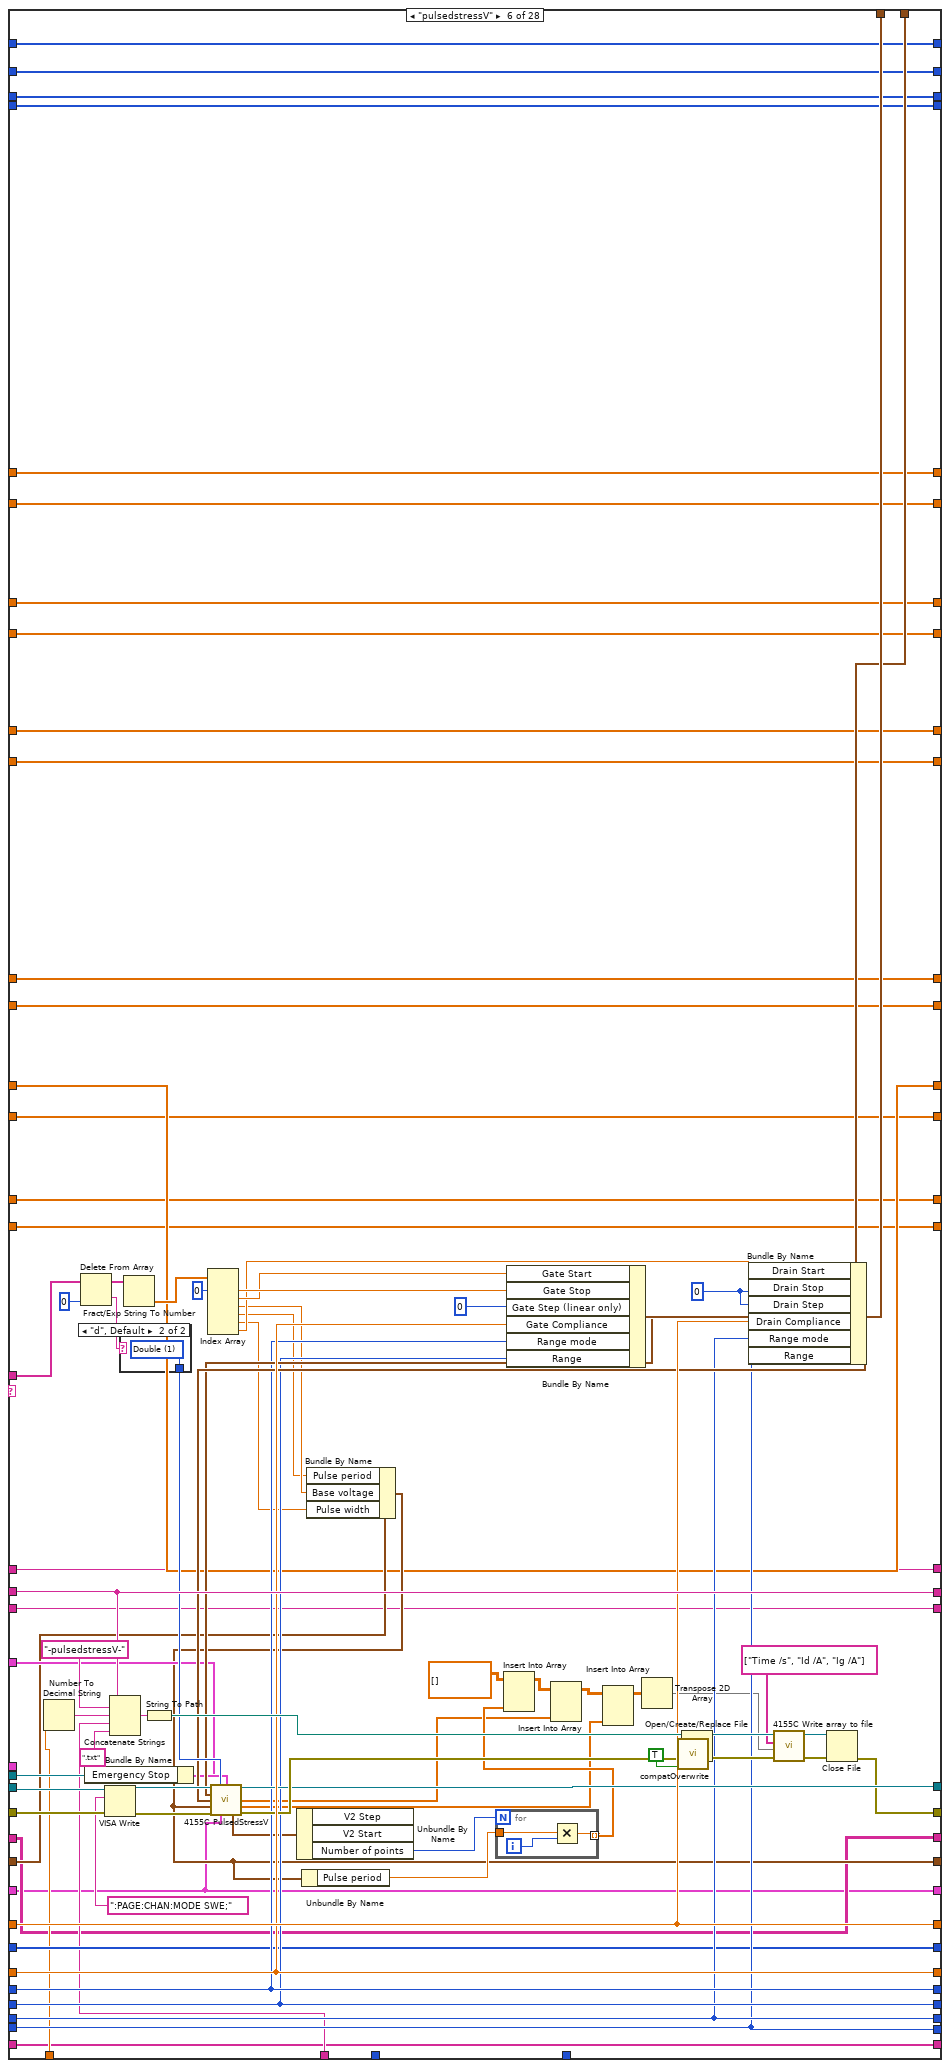
[diagram p14: hidden frame]
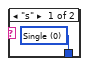
[diagram p15: hidden frame]
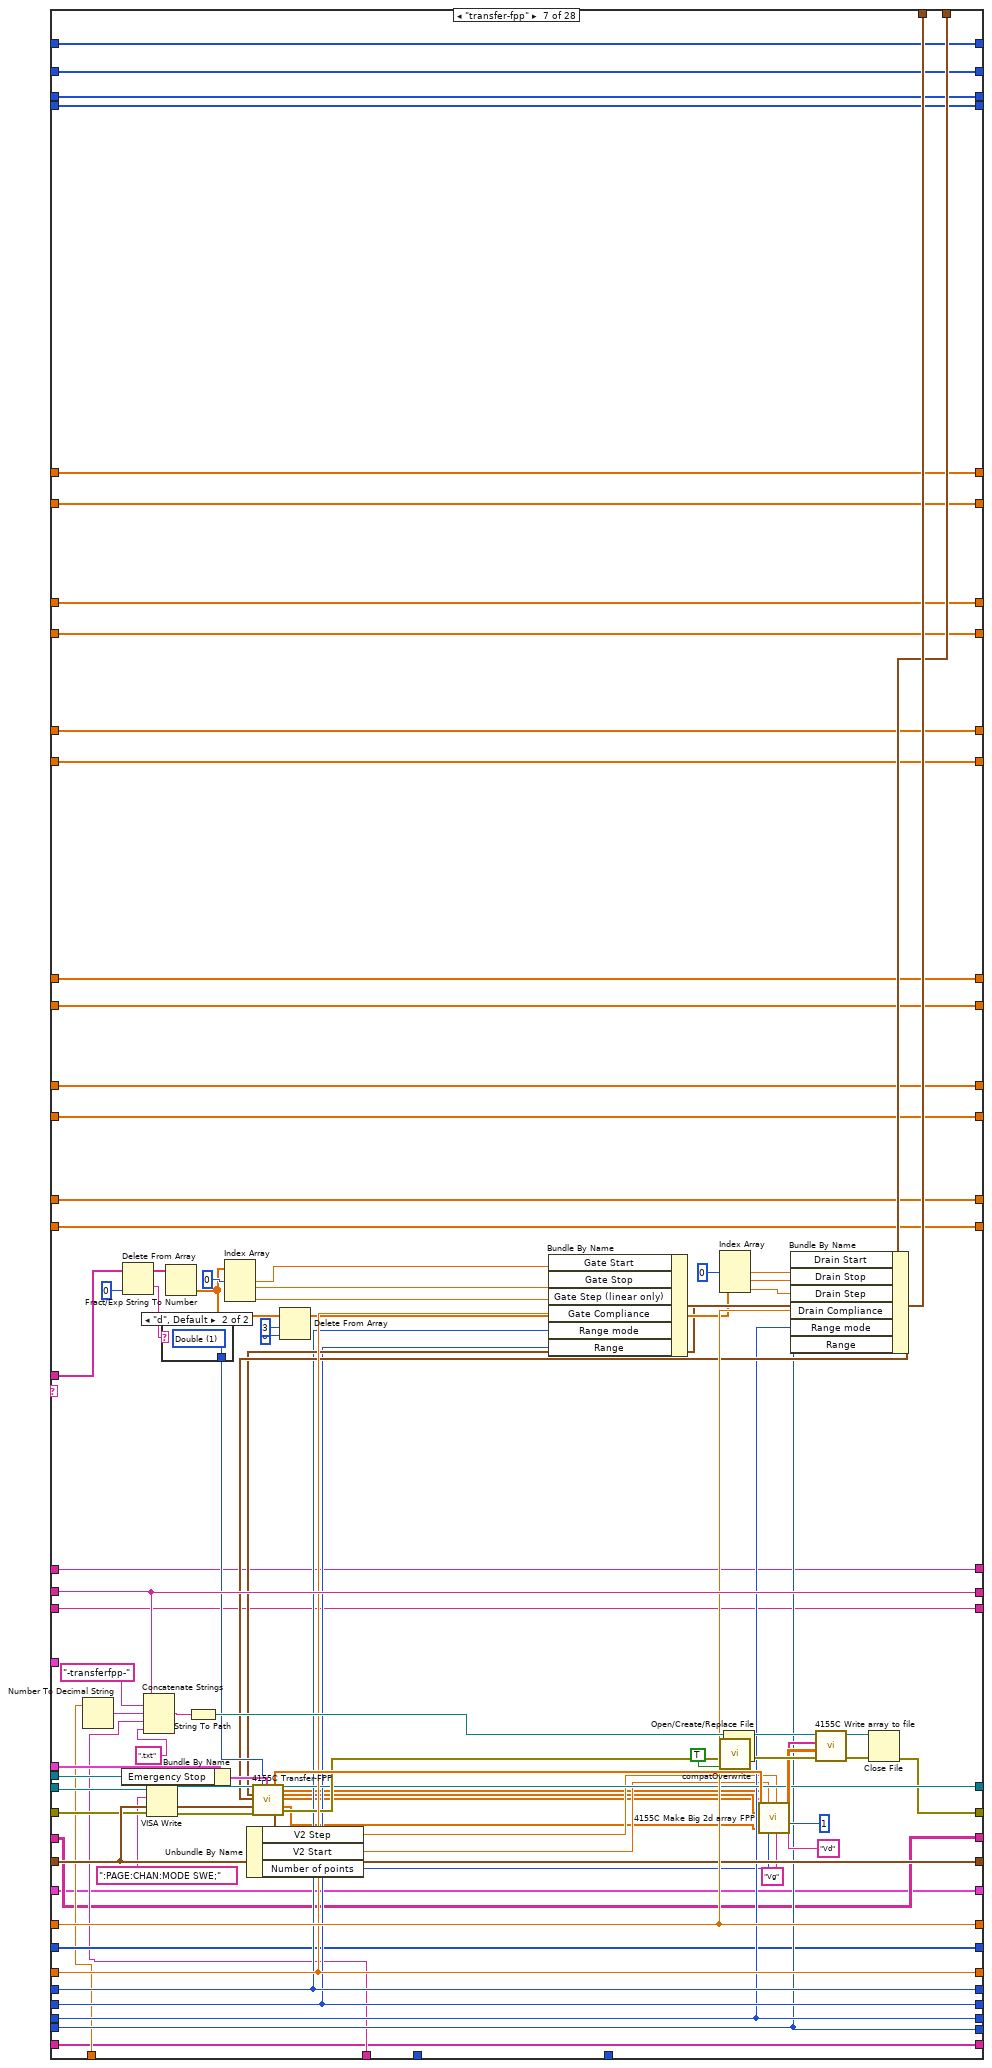
[diagram p16: hidden frame]
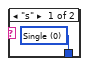
[diagram p17: hidden frame]
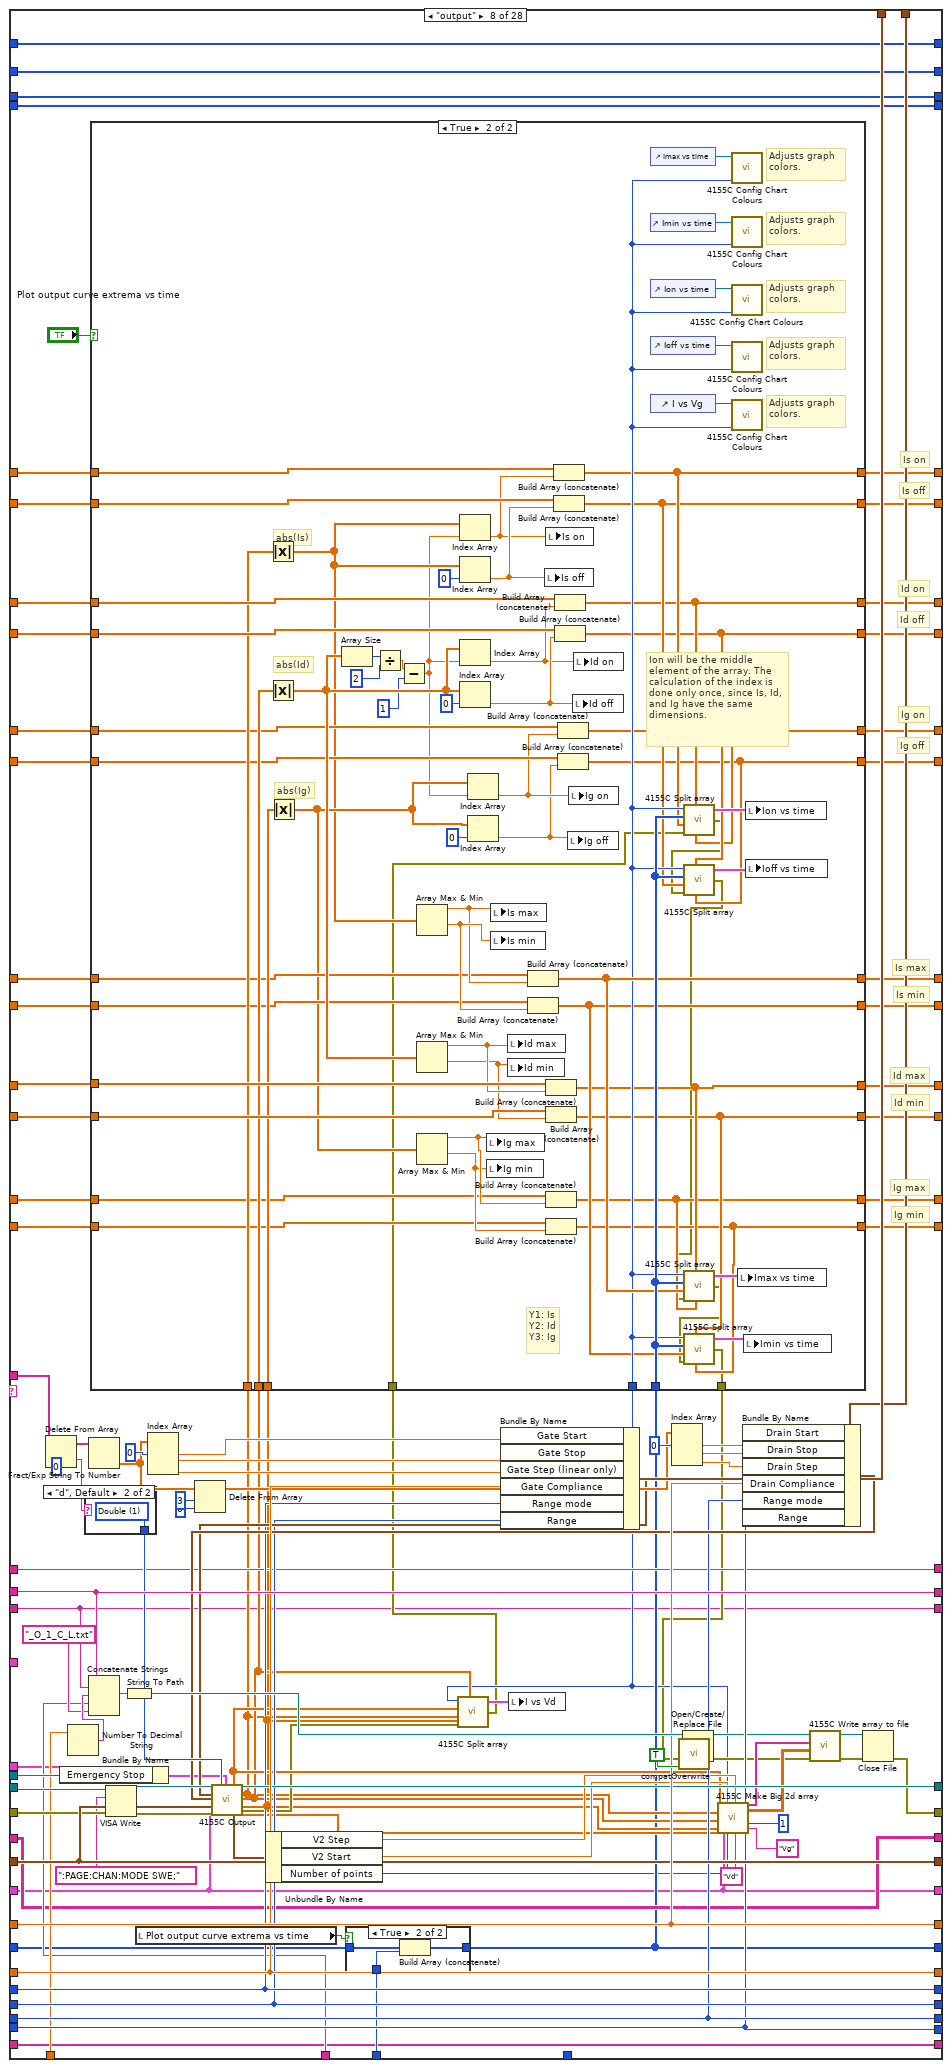
[diagram p18: hidden frame]
diagram:
  w10 = cluster{"Y data in":dbl[], "X data in":dbl[]}[] [] ("I vs Vg")
  w11 = 0.0 ("Is off")
  w12 = 0.0 ("Is on")
  w13 = 0.0 ("Is min")
  w14 = 0.0 ("Is max")
  w63 = u16 1 items=["Reset All", "Partial reset"] ("Type of reset")
  # "Change from previous version:\n\n- Added SMU4 command."
  # "This is a version specific to the SPM pump."
  # "I add 1 to both the \"total lines\" and the \"line running\" indicators because i and N begin from 0, and the script lines begin from 1."
  # "Bugs:\n\n- If using the \"filename\" command, keep in mind that the arrays of the time-dependent data are not re-initialized inbetween filename changes. \n\n- Do not connect the \"error\" wire of a Split block if it has unconnected terminals! It will halt the program."
  # "Array size"
  # "%s option converts a spreadsheet string to an array of strings."
  # "0: No of rows of array\n1: No of cols"
  # "Dimitrios Simatos\nv. 6.5"
  # "Changes from original textcontrol.vi:\n\n- Timestamp appears in filename.\n- (Only) transfer and output curves are plotted.\n- Communication with serial port.\n- Can execute any command, as all pattern matching functions were replaced. Previously, commands with special LabVIEW characters could not be executed.\n- Replaced write to file function with write to text file.\n- Replaced while loop with for loop.\n- Replaced 4155C \"Save File\" function and now the vi can save time-dependent variables.\n- Added clock with start time control and various units.\n- Changed filepath in which the program is saved.\n- Added a serial output log that keeps a history.\n- Tab control.\n- Addition of specialized serial read/write file for the SPM OEM pump.\n- Added halt and hard stop.\n- Added option for plotting transfer and output curve extrema vs time.\n- Corrected bug of \"itime\" command. The command did not allow for settting the integration time value, it allowed to set the category of the integration time (short, medium, long). If the time value was beyond the range of the category, then the SPA used the closest value allowed, whilst staying in the category. So, if the integration time was changed to long, but the integration time value was a short one, then the SPA would measure using the minimum long integration time value and not the value that the user intended."
  # "Search and replace LF with EOL"
  n1 = Equal?(x="integration time", y=u32 0) -> (x = y?=w64:bool)
  n2 = Select(t="Integration time (short)", s=w64, f="Integration time (long)") -> (s? t:f=w15:dbl)
  n3 = call "4155C Get Filename.vi"("error in (no error)"=errorcluster {"status"=FALSE, "code"=0, "source"=""}) -> ("error out"=w58:errorcluster, "path"=w33:path)  [unwired: 2 in, 1 out]
  "Path" <- w33
  n4 = Bundle By Name(cluster="Timings (overwritten by the Front Panel)", "integration time"="integration time", "Short/Long integration time"=w15) -> (w56:T5)
  n5 = Path To String(path=w33) -> (string=w34:string)
  n6 = Search and Replace String(replace all?=TRUE ("replace all? (F)"), input string="Script", search string="\n", replace string="\r\n") -> (result string=w46:string)  [unwired: 4 in, 3 out]
  n7 = Match Pattern(string=w34, regular expression=".txt") -> (before substring=w29:string)  [unwired: 1 in, 3 out]
  n8 = call "4155C Initialise.vi"("VISA resource name in"=refnum<visa-resource-name> "GPIB0::14::INSTR", "Reset"="Full Reset", "Type of reset"=w63, "error in (no error)"=w58, "VISA Timeout Value"=u32 10000) -> ("VISA Resource Name out"=w57:refnum<visa-resource-name>, "error out"=w3:errorcluster)
  n9 = Concatenate Strings(w29, "Suffix (script)") -> (w28:string)
  n10 = Spreadsheet String To Array(delimiter (Tab)="\r\n", format string="%s", spreadsheet string="Script", array type (2D Dbl)="") -> (array=w37:string[][])
  n11 = String To Path(string=w28) -> (path=w6:path)
  n12 = Array Size(array=w37) -> (size(s)=w41:i32[])
  n13 = Initialize Array("") -> (w20:string[])  [unwired: 1 in]
  n14 = Open/Create/Replace File(file path (use dialog)=w6, error in=w3, operation (0:open)=T8."replace or create with confirmation") -> (refnum out=w5:refnum<file>, error out=w4:errorcluster)  [unwired: 3 in, 1 out]
  n15 = Initialize Array(0 ("element")) -> (w22:i32[])  [unwired: 1 in]
  n16 = Initialize Array("") -> (w18:string[][])  [unwired: 2 in]
  n17 = Initialize Array(0.0 ("element")) -> (w24:dbl[])  [unwired: 1 in]
  n18 = Index Array(array=w41, index=0) -> (element=w39:i32)
  n19 = Write to Text File(file (use dialog)=w5, text=w46, error in=w4) -> (error out=w27:errorcluster)  [unwired: 1 in, 2 out]
  n20 = for {
    N: w39 -> [w180]
    shift-left: "Source/Drain Range" -> [w221]
    shift-right: [w217] -> _
    shift-left: "Source/Drain\nRange mode" -> [w222]
    shift-right: [w218] -> _
    shift-left: "Gate Range" -> [w223]
    shift-right: [w219] -> _
    shift-left: "Gate Range\nmode" -> [w224]
    shift-right: [w220] -> _
    shift-left: "Gate: Compliance" -> [w233]
    shift-right: [w229] -> _
    shift-left: "Drain: Compliance" -> [w234]
    shift-right: [w230] -> _
    shift-left: w56 -> [w235]
    shift-right: [w231] -> w16
    shift-left: w27 -> [w236]
    shift-right: [w126] -> w32
    shift-left: w57 -> [w237]
    shift-right: [w232] -> _
    shift-left: w29 -> [w238]
    shift-right: [w130] -> _
    tunnel: "Panel Controls 2" -> [w215]
    shift-right: [w88] -> _
    shift-left: w24 -> [w214]
    shift-right: [w150] -> _
    shift-left: i32[] [] -> [w210]
    tunnel: w37 -> [w209] mode=indexing
    shift-right: [w87] -> _
    shift-left: w24 -> [w186]
    shift-right: [w120] -> _
    shift-left: w20 -> [w172]
    shift-right: [w151] -> _
    shift-left: w22 -> [w167]
    shift-right: [w132] -> _
    shift-left: w22 -> [w166]
    shift-right: [w165] -> _
    shift-left: "" -> [w164]
    shift-right: [w125] -> _
    shift-left: w22 -> [w147]
    shift-right: [w124] -> _
    shift-left: w22 -> [w131]
    shift-right: [w121] -> _
    shift-left: w18 -> [w123]
    shift-right: [w81] -> _
    shift-left: w24 -> [w109]
    shift-right: [w82] -> _
    shift-left: w24 -> [w108]
    shift-right: [w86] -> _
    shift-left: w24 -> [w97]
    shift-right: [w85] -> _
    shift-left: w24 -> [w96]
    shift-right: [w79] -> _
    shift-left: w24 -> [w95]
    shift-right: [w89] -> _
    shift-left: w24 -> [w94]
    shift-right: [w80] -> _
    shift-left: w24 -> [w93]
    shift-right: [w78] -> _
    shift-left: w24 -> [w92]
    shift-right: [w84] -> _
    shift-left: w24 -> [w91]
    shift-right: [w83] -> _
    shift-left: w24 -> [w90]
    shift-right: [w73] -> _
    shift-left: "Filename (variable part)" -> [w72]
    shift-right: [w69] -> w1
    shift-left: "SMU4" -> [w216]
    i -> [w175]
    stop <- "Interrupt program" stop-if-true
    # "Filename prefix"
    # "Is off"
    # "Is on"
    # "Ig off"
    # "Ig on"
    # "Is min"
    # "Is max"
    # "Ig min"
    # "Ig max"
    # "Id min"
    # "Id max"
    # "Id off"
    # "Id on"
    # "Pump status"
    # "Filepath and name"
    # "Pump status"
    # "Limit of command arguments (array columns). Raise if needed."
    # "Serial port data (string)"
    # "Serial port data (table)"
    # "Time array for valve position"
    # "Time array for absolute plunger position"
    # "Valve position"
    # "Absolute plunger position"
    # "Serial port data"
    # "For loop counter"
    # "<-----Equivalent to the 4155C \"Write\" subvi.----->"
    # "Headers"
    # "Save transfer curves in file."
    # "Filepath and name"
    # "Save time-dependent data."
    # "Use the time offset if your measurements do not start at t=0."
    # "Time for Imax, Imin, Ion, Ioff"
    # "Rest of elements of command"
    # "First element of command\n(case select)"
    n21 = Add(x=w175, y=1) -> (x+y=→"Line running":i32)
    n22 = Add(x=w180, y=1) -> (x+y=→"Total lines":i32)
    n23 = Index Array(array=w209, index=0 ("line index")) -> (element=w204:string)
    "Command running:" <- w204
    n24 = control-ref of="Interrupt scan"() -> (w228:refnum<vi>)
    n25 = Spreadsheet String To Array(delimiter (Tab)=" ", format string="%s", spreadsheet string=w204, array type (2D Dbl)=string[] []) -> (array=w202:string[])
    n26 = Delete From Array(array=w202, index=0) -> (deleted portion=w110:string, array with subset deleted=w201:string[])  [unwired: 1 in]
    n27 = call "Elapsed Time"("Reset"="Reset", "Auto Reset"="Auto Reset") -> ("Elapsed Time (s)"=w211:dbl)  [unwired: 10 in, 7 out]
    n28 = case shown="0, Default" "Time Units" {
      tunnel: ["_sec" "_min" "_h"] -> w212
      tunnel: [w242 w246 w249] -> w182
      tunnel: w211 -> [w242 w245 w250]
      frame 0, Default {
      }
      frame 1 {
        n29 = Divide(x=w245, y=60.0) -> (x/y=w246:dbl)
      }
      frame 2 {
        n30 = Divide(x=w250, y=3600.0) -> (x/y=w249:dbl)
      }
    }
    n31 = Add(x=w182, y="Time Offset") -> (x+y=w181:dbl)
    n32 = To Long Integer(number=w181) -> (32bit integer=w148:i32)
    "Elapsed Time" <- w148
    n33 = case shown="\"SMU4\"" w110 {
      tunnel: w201 -> [w288 w327 w365 w369 w505 w613 w759 w879 w1041 w1069 w1150 w1197 w1242 w1283 w1317 _ _ w1481 w1562 _ w1667 w1731 w1793 w1883 w1965 w2005 w2076 w2131]
      tunnel: w238 -> [w283 w323 w363 w391 w512 w677 w767 w886 w1049 w1092 w1139 w1189 w1235 w1277 w1310 w1349 w1411 w1459 w1544 w1595 w1654 w1718 w1781 w1877 w1961 w2007 w2078 w2133]
      tunnel: w237 -> [w282 w322 w354 w389 w483 w662 w736 w857 w1017 w1093 w1140 w1190 w1236 w1278 w1311 w1354 w1413 w1487 w1568 w1599 w1673 w1737 w1799 w1889 w1919 w2011 w2082 w2135]
      tunnel: w236 -> [w281 w321 w353 w388 w482 w661 w735 w856 w1014 w1094 w1141 w1191 w1237 w1279 w1312 w1353 w1384 w1486 w1567 w1598 w1672 w1736 w1798 w1888 w1918 w2010 w2081 w2136]
      tunnel: w235 -> [w280 w320 w362 w386 w508 w638 w763 w882 w1045 w1102 w1149 w1188 w1234 w1276 w1309 w1352 w1408 w1450 w1536 w1604 w1647 w1711 w1774 w1876 w1960 w2012 w2083 w2138]
      tunnel: w234 -> [w279 w319 w361 w385 w510 w675 w765 w884 w1047 w1101 w1148 w1196 w1241 w1282 w1316 w1351 w1393 w1485 w1566 w1607 w1671 w1735 w1797 w1887 w1969 w2013 w2084 w2139]
      tunnel: w233 -> [w278 w318 w360 w383 w509 w674 w764 w883 w1046 w1100 w1147 w1195 w1240 w1281 w1315 w1350 w1394 w1460 w1545 w1606 w1655 w1719 w1782 w1878 w1962 w2015 w2085 w2141]
      tunnel: [w282 w322 w352 w389 w507 w672 w761 w881 w1043 w1093 w1140 w1190 w1236 w1278 w1311 w1354 w1413 w1451 w1518 w1597 w1648 w1712 w1775 w1829 w1921 w2011 w2082 w2135] -> w232
      tunnel: [w281 w321 w351 w388 w506 w671 w760 w880 w1042 w1094 w1141 w1191 w1237 w1279 w1312 w1353 w1383 w1461 w1519 w1596 w1656 w1720 w1783 w1828 w1920 w2009 w2080 w2136] -> w146
      tunnel: [w280 w320 w362 w386 w508 w634 w763 w882 w1045 w1095 w1142 w1188 w1234 w1276 w1309 w1352 w1408 w1450 w1536 w1604 w1647 w1711 w1774 w1876 w1960 w2012 w2083 w2138] -> w231
      tunnel: [w279 w319 w361 w385 w510 w675 w765 w884 w1047 w1101 w1148 w1196 w1241 w1282 w1316 w1351 w1393 w1485 w1566 w1607 w1671 w1735 w1797 w1887 w1969 w2013 w2084 w2139] -> w230
      tunnel: [w278 w318 w360 w383 w509 w674 w764 w883 w1046 w1100 w1147 w1195 w1240 w1281 w1315 w1350 w1394 w1460 w1545 w1606 w1655 w1719 w1782 w1878 w1962 w2015 w2085 w2141] -> w229
      tunnel: [w283 w323 w363 w391 w512 w677 w767 w886 w1049 w1092 w1139 w1189 w1235 w1277 w1310 w1349 w1411 w1459 w1544 w1595 w1654 w1718 w1781 w1877 w1961 w2007 w2078 w2133] -> w130
      tunnel: w228 -> [_ _ _ _ w514 w681 w772 w888 w1053 _ _ _ _ _ _ _ _ w1456 w1541 _ w1653 w1717 w1780 w1849 w1937 _ _ _]
      tunnel: "Gate" -> [_ _ _ _ w492 w665 w746 w866 w1028 _ _ _ _ _ _ _ _ _ _ _ _ _ _ _ _ _ _ _]
      tunnel: "Drain 2" -> [_ _ _ _ w491 w664 w745 w865 w1027 _ _ _ _ _ _ _ _ _ _ _ _ _ _ _ _ _ _ _]
      tunnel: "Panel Controls" -> [_ _ _ _ _ _ w744 w786 w1026 _ _ _ _ _ _ _ _ _ _ _ _ _ _ _ _ _ _ _]
      tunnel: w224 -> [w277 w317 w359 w382 w476 w655 w729 w850 w1012 w1099 w1146 _ w1233 w1275 w1308 w1348 w1395 w1446 w1532 w1600 w1643 w1707 w1770 w1872 w1956 w2016 w2086 w2142]
      tunnel: w223 -> [w276 w316 w358 w381 w475 w654 w728 w849 w1011 w1098 w1145 w1194 _ w1266 w1314 w1347 w1396 w1447 w1533 w1601 w1644 w1708 w1771 w1873 w1957 w2017 w2087 w2143]
      tunnel: w222 -> [w275 w315 w357 w380 w474 w653 w727 w848 w1010 w1097 w1144 w1193 w1239 w1280 _ w1346 w1397 w1448 w1534 w1602 w1645 w1709 w1772 w1874 w1958 w2018 w2088 w2144]
      tunnel: w221 -> [w274 w314 w356 w379 w473 w652 w726 w847 w1013 w1096 w1143 w1192 w1238 _ w1313 w1345 w1398 w1449 w1535 w1603 w1646 w1710 w1773 w1875 w1959 w2019 w2089 w2145]
      tunnel: [w277 w317 w359 w382 w476 w655 w729 w850 w1012 w1099 w1146 w1187 w1233 w1275 w1308 w1348 w1395 w1446 w1532 w1600 w1643 w1707 w1770 w1872 w1956 w2016 w2086 w2142] -> w220
      tunnel: [w276 w316 w358 w381 w475 w654 w728 w849 w1011 w1098 w1145 w1194 w1225 w1266 w1314 w1347 w1396 w1447 w1533 w1601 w1644 w1708 w1771 w1873 w1957 w2017 w2087 w2143] -> w219
      tunnel: [w275 w315 w357 w380 w474 w653 w727 w848 w1010 w1097 w1144 w1193 w1239 w1280 w1307 w1346 w1397 w1448 w1534 w1602 w1645 w1709 w1772 w1874 w1958 w2018 w2088 w2144] -> w218
      tunnel: [w274 w314 w356 w379 w473 w652 w726 w847 w1013 w1096 w1143 w1192 w1238 w1267 w1313 w1345 w1398 w1449 w1535 w1603 w1646 w1710 w1773 w1875 w1959 w2019 w2089 w2145] -> w217
      tunnel: w216 -> [w252 w289 w328 _ w409 w601 w692 w783 w975 w1066 w1116 w1165 w1203 w1244 w1285 w1323 w1355 w1414 w1492 w1573 w1608 w1676 w1740 w1802 w1890 w1970 w2020 w2129]
      tunnel: w215 -> [_ _ _ _ w467 w649 _ _ _ _ _ _ _ _ _ _ _ _ _ _ _ _ _ _ _ _ _ _]
      tunnel: [w273 w310 w349 w396 w424 w626 w716 w799 w999 w1091 w1137 w1186 w1224 w1265 w1306 w1344 w1379 w1438 w1497 w1594 w1632 w1700 w1764 w1826 w1914 w2008 w2079 w2150] -> w88
      tunnel: w214 -> [w273 w310 w349 w396 w464 w626 w716 w839 w999 w1091 w1137 w1186 w1224 w1265 w1306 w1344 w1379 w1438 w1497 w1594 w1632 w1700 w1764 w1826 w1914 w2008 w2079 w2150]
      tunnel: w181 -> [_ _ _ _ w463 w623 w714 w838 w996 _ _ _ _ _ _ _ w1377 w1436 w1514 _ w1629 w1697 w1761 w1823 w1910 _ _ _]
      tunnel: w212 -> [_ _ _ _ w460 w622 w712 w835 w995 _ _ _ _ _ _ _ w1375 w1434 w1513 _ w1628 w1696 w1760 w1822 w1911 _ w2047 _]
      tunnel: w148 -> [_ _ _ _ w456 _ _ w831 _ _ _ _ _ _ _ _ _ _ _ _ _ _ _ _ _ _ w2050 _]
      tunnel: [w272 w309 w348 w384 w428 w625 w715 w803 w998 w1090 w1136 w1185 w1223 w1264 w1305 w1343 w1378 w1437 w1516 w1593 w1631 w1699 w1763 w1825 w1913 w2014 w2059 w2140] -> w150
      tunnel: w210 -> [w272 w309 w348 w384 w459 w625 w715 w834 w998 w1090 w1136 w1185 w1223 w1264 w1305 w1343 w1378 w1437 w1516 w1593 w1631 w1699 w1763 w1825 w1913 w2014 w2059 w2140]
      tunnel: [w271 w308 w347 w395 w423 w621 w711 w798 w994 w1089 w1135 w1184 w1222 w1263 w1304 w1342 w1374 w1433 w1496 w1592 w1627 w1695 w1759 w1821 w1909 w2003 w2075 w2149] -> w87
      tunnel: w186 -> [w271 w308 w347 w395 w455 w621 w711 w830 w994 w1089 w1135 w1184 w1222 w1263 w1304 w1342 w1374 w1433 w1496 w1592 w1627 w1695 w1759 w1821 w1909 w2003 w2075 w2149]
      tunnel: [w270 w307 w346 w378 w448 w620 w710 w823 w993 w1088 w1134 w1183 w1221 w1262 w1303 w1341 w1373 w1432 w1512 w1591 w1626 w1694 w1758 w1820 w1908 w2002 w2074 w2146] -> w120
      tunnel: w172 -> [w270 w307 w346 w378 w448 w620 w710 w823 w993 w1088 w1134 w1183 w1221 w1262 w1303 w1341 w1373 w1432 w1512 w1591 w1626 w1694 w1758 w1820 w1908 w2001 w2048 w2146]
      tunnel: [w269 w306 w345 w406 w447 w619 w709 w822 w992 w1087 w1133 w1182 w1220 w1261 w1302 w1340 w1372 w1431 w1511 w1590 w1625 w1693 w1757 w1819 w1907 w1987 w2061 w2160] -> w151
      tunnel: w167 -> [w269 w306 w345 w406 w447 w619 w709 w822 w992 w1087 w1133 w1182 w1220 w1261 w1302 w1340 w1372 w1431 w1511 w1590 w1625 w1693 w1757 w1819 w1907 w1987 w2060 w2160]
      tunnel: [w268 w305 w344 w408 w446 w618 w708 w821 w991 w1086 w1132 w1181 w1219 w1260 w1301 w1339 w1371 w1430 w1510 w1589 w1624 w1692 w1756 w1818 w1906 w1986 w2043 w2162] -> w132
      tunnel: w166 -> [w268 w305 w344 w408 w446 w618 w708 w821 w991 w1086 w1132 w1181 w1219 w1260 w1301 w1339 w1371 w1430 w1510 w1589 w1624 w1692 w1756 w1818 w1906 w1986 w2041 w2162]
      tunnel: [w267 w304 w343 w392 w445 w617 w707 w820 w990 w1085 w1131 w1180 w1218 w1259 w1300 w1338 w1370 w1429 w1509 w1588 w1623 w1691 w1755 w1817 w1905 w1985 w2040 w2134] -> w165
      tunnel: w164 -> [w267 w304 w343 w392 w445 w617 w707 w820 w990 w1085 w1131 w1180 w1218 w1259 w1300 w1338 w1370 w1429 w1509 w1588 w1623 w1691 w1755 w1817 w1905 w1985 w2051 w2134]
      tunnel: w148 -> [_ _ _ _ _ _ _ _ _ _ _ _ _ _ _ _ _ _ _ _ _ _ _ _ _ _ w2039 _]
      tunnel: w147 -> [w266 w303 w342 w407 w444 w616 w706 w819 w989 w1084 w1130 w1179 w1217 w1258 w1299 w1337 w1369 w1428 w1508 w1587 w1622 w1690 w1754 w1816 w1904 w1984 w2038 w2161]
      tunnel: [w266 w303 w342 w407 w444 w616 w706 w819 w989 w1084 w1130 w1179 w1217 w1258 w1299 w1337 w1369 w1428 w1508 w1587 w1622 w1690 w1754 w1816 w1904 w1984 w2037 w2161] -> w125
      tunnel: [w265 w302 w341 w405 w443 w615 w705 w818 w988 w1083 w1129 w1178 w1216 w1257 w1298 w1336 w1368 w1427 w1507 w1586 w1621 w1689 w1753 w1815 w1903 w1983 w2036 w2159] -> w124
      tunnel: w131 -> [w265 w302 w341 w405 w443 w615 w705 w818 w988 w1083 w1129 w1178 w1216 w1257 w1298 w1336 w1368 w1427 w1507 w1586 w1621 w1689 w1753 w1815 w1903 w1983 w2035 w2159]
      tunnel: [w264 w301 w340 w387 w442 w614 w704 w817 w987 w1082 w1128 w1177 w1215 w1256 w1297 w1335 w1367 w1426 w1506 w1585 w1620 w1688 w1752 w1814 w1902 w1982 w2033 w2137] -> w121
      tunnel: w123 -> [w264 w301 w340 w387 w442 w614 w704 w817 w987 w1082 w1128 w1177 w1215 w1256 w1297 w1335 w1367 w1426 w1506 w1585 w1620 w1688 w1752 w1814 w1902 w1982 w2032 w2137]
      tunnel: [w262 w299 w338 w401 w417 w611 w702 w792 w985 w1080 w1127 w1176 w1213 w1254 w1295 w1333 w1365 w1425 w1505 w1584 w1619 w1687 w1750 w1813 w1901 w1981 w2031 w2155] -> w81
      tunnel: w109 -> [w262 w299 w338 w401 w441 w611 w702 w816 w985 w1080 w1127 w1176 w1213 w1254 w1295 w1333 w1365 w1425 w1505 w1584 w1619 w1687 w1750 w1813 w1901 w1981 w2031 w2155]
      tunnel: [w263 w300 w339 w402 w418 w612 w703 w793 w986 w1081 w1126 w1175 w1214 w1255 w1296 w1334 w1366 w1424 w1504 w1583 w1618 w1686 w1751 w1812 w1900 w1980 w2030 w2156] -> w82
      tunnel: w108 -> [w263 w300 w339 w402 w440 w612 w703 w815 w986 w1081 w1126 w1175 w1214 w1255 w1296 w1334 w1366 w1424 w1504 w1583 w1618 w1686 w1751 w1812 w1900 w1980 w2030 w2156]
      tunnel: [w255 w292 w331 w394 w422 w608 w700 w797 w983 w1073 w1124 w1173 w1211 w1252 w1293 w1331 w1358 w1417 w1495 w1582 w1611 w1679 w1743 w1805 w1895 w1973 w2029 w2148] -> w86
      tunnel: w97 -> [w255 w292 w331 w394 w436 w608 w700 w811 w983 w1073 w1124 w1173 w1211 w1252 w1293 w1331 w1358 w1417 w1495 w1582 w1611 w1679 w1743 w1805 w1895 w1973 w2029 w2148]
      tunnel: [w254 w291 w330 w393 w421 w609 w701 w796 w984 w1072 w1125 w1174 w1212 w1253 w1294 w1332 w1357 w1416 w1494 w1581 w1610 w1678 w1742 w1804 w1894 w1972 w2028 w2147] -> w85
      tunnel: w96 -> [w254 w291 w330 w393 w435 w609 w701 w810 w984 w1072 w1125 w1174 w1212 w1253 w1294 w1332 w1357 w1416 w1494 w1581 w1610 w1678 w1742 w1804 w1894 w1972 w2028 w2147]
      tunnel: [w257 w294 w333 w398 w427 w607 w698 w802 w981 w1078 w1122 w1171 w1209 w1250 w1291 w1329 w1360 w1419 w1499 w1576 w1613 w1681 w1745 w1807 w1893 w1977 w2026 w2152] -> w79
      tunnel: w95 -> [w257 w294 w333 w398 w434 w607 w698 w809 w981 w1078 w1122 w1171 w1209 w1250 w1291 w1329 w1360 w1419 w1499 w1576 w1613 w1681 w1745 w1807 w1893 w1977 w2026 w2152]
      tunnel: [w256 w293 w332 w397 w425 w610 w699 w800 w982 w1079 w1123 w1172 w1210 w1251 w1292 w1330 w1359 w1418 w1498 w1575 w1612 w1680 w1744 w1806 w1892 w1976 w2027 w2151] -> w89
      tunnel: w94 -> [w256 w293 w332 w397 w433 w610 w699 w808 w982 w1079 w1123 w1172 w1210 w1251 w1292 w1330 w1359 w1418 w1498 w1575 w1612 w1680 w1744 w1806 w1892 w1976 w2027 w2151]
      tunnel: [w259 w296 w335 w400 w416 w606 w696 w791 w979 w1076 w1120 w1169 w1207 w1248 w1289 w1327 w1362 w1421 w1501 w1578 w1615 w1683 w1747 w1809 w1897 w1979 w2024 w2154] -> w80
      tunnel: w93 -> [w259 w296 w335 w400 w432 w606 w696 w807 w979 w1076 w1120 w1169 w1207 w1248 w1289 w1327 w1362 w1421 w1501 w1578 w1615 w1683 w1747 w1809 w1897 w1979 w2024 w2154]
      tunnel: [w258 w295 w334 w399 w415 w605 w697 w790 w980 w1077 w1121 w1170 w1208 w1249 w1290 w1328 w1361 w1420 w1500 w1577 w1614 w1682 w1746 w1808 w1896 w1978 w2025 w2153] -> w78
      tunnel: w92 -> [w258 w295 w334 w399 w431 w605 w697 w806 w980 w1077 w1121 w1170 w1208 w1249 w1290 w1328 w1361 w1420 w1500 w1577 w1614 w1682 w1746 w1808 w1896 w1978 w2025 w2153]
      tunnel: [w261 w298 w337 w404 w420 w604 w694 w795 w977 w1074 w1118 w1167 w1205 w1246 w1287 w1325 w1364 w1423 w1503 w1580 w1617 w1685 w1749 w1811 w1899 w1975 w2022 w2158] -> w84
      tunnel: w91 -> [w261 w298 w337 w404 w430 w604 w694 w805 w977 w1074 w1118 w1167 w1205 w1246 w1287 w1325 w1364 w1423 w1503 w1580 w1617 w1685 w1749 w1811 w1899 w1975 w2022 w2158]
      tunnel: [w260 w297 w336 w403 w419 w603 w695 w794 w978 w1075 w1119 w1168 w1206 w1247 w1288 w1326 w1363 w1422 w1502 w1579 w1616 w1684 w1748 w1810 w1898 w1974 w2023 w2157] -> w83
      tunnel: w90 -> [w260 w297 w336 w403 w429 w603 w695 w804 w978 w1075 w1119 w1168 w1206 w1247 w1288 w1326 w1363 w1422 w1502 w1579 w1616 w1684 w1748 w1810 w1898 w1974 w2023 w2157]
      tunnel: w72 -> [w253 w290 w329 w390 w412 w602 w693 w787 w976 w1071 w1117 w1166 w1204 w1245 w1286 w1324 w1356 w1415 w1493 w1574 w1609 w1677 w1741 w1803 w1891 w1971 w2021 _]
      tunnel: [w253 w290 w329 w390 w412 w602 w693 w787 w976 w1071 w1117 w1166 w1204 w1245 w1286 w1324 w1356 w1415 w1493 w1574 w1609 w1677 w1741 w1803 w1891 w1971 w2021 w2130] -> w73
      tunnel: [w252 w289 w328 w368 w409 w601 w692 w783 w975 w1066 w1116 w1165 w1203 w1244 w1285 w1323 w1355 w1414 w1492 w1573 w1608 w1676 w1740 w1802 w1890 w1970 w2020 w2129] -> w69
      frame "wait" {
        n34 = Index Array(array=w288, index=0 ("Index")) -> (element=w286:string)
        n35 = Decimal String To Number(string=w286, default (0L)=u32 0) -> (number=w285:u32)  [unwired: 1 in, 1 out]
        n36 = Wait (ms)(milliseconds to wait=w285) -> ()  [unwired: 1 out]
      }
      frame "wait-min" {
        n37 = Index Array(array=w327, index=0 ("Index")) -> (element=w325:string)
        n38 = Decimal String To Number(string=w325, default (0L)=u32 0) -> (number=w313:u32)  [unwired: 1 in, 1 out]
        n39 = Multiply(x=w313, y=u32 60000) -> (x*y=w312:u32)
        n40 = Wait (ms)(milliseconds to wait=w312) -> ()  [unwired: 1 out]
      }
      frame "standby" {
        n41 = Index Array(array=w365, index=0 ("Index")) -> (element=w355:string)
        n42 = case shown="\"off\", Default" w355 {
          tunnel: [":PAGE:SCON:STAN 0" ":PAGE:SCON:STAN 1"] -> w350
          frame "off", Default {
          }
          frame "on" {
          }
        }
        n43 = VISA Write(VISA resource name=w354, write buffer=w350, error in (no error)=w353) -> (VISA resource name out=w352:refnum<visa-resource-name>, error out=w351:errorcluster)  [unwired: 1 out]
      }
      frame "SMU4" {
        n44 = Delete From Array(array=w369, index=0) -> (deleted portion=w372:string, array with subset deleted=w375:string[])  [unwired: 1 in]
        n45 = Equal?(x=w372, y="ON") -> (x = y?=w370:bool)
        n46 = Delete From Array(array=w375, index=0) -> (deleted portion=w374:string)  [unwired: 1 in, 1 out]
        n47 = Fract/Exp String To Number(string=w374) -> (number=w371:dbl)  [unwired: 3 in, 1 out]
        n48 = Bundle(w370, w371) -> (w368:cluster{bool, dbl})  [unwired: 1 in]
      }
      frame "transfer" {
        # "Is off"
        # "Is on"
        # "Ig off"
        # "Ig on"
        # "Is min"
        # "Is max"
        # "Ig min"
        # "Ig max"
        # "Id min"
        # "Id max"
        # "Id off"
        # "Id on"
        n49 = Delete From Array(array=w505, index=0 ("Index")) -> (deleted portion=w503:string, array with subset deleted=w502:string[])  [unwired: 1 in]
        n50 = Bundle By Name(cluster=w467, "Emergency Stop"=w514) -> (w468:T2)
        n51 = Number To Decimal String(number=w463) -> (decimal integer string=w462:string)  [unwired: 1 in]
        n52 = case shown="\"d\", Default" w503 {
          tunnel: [w599 w600] -> w501
          frame "s" {
            w599 = u16 0 items=["Single", "Double"] ("sweep mode")
          }
          frame "d", Default {
            w600 = u16 1 items=["Single", "Double"] ("sweep mode")
          }
        }
        n53 = Fract/Exp String To Number(string=w502) -> (number=w487:dbl[])  [unwired: 3 in, 1 out]
        n54 = Concatenate Strings(w512, w412, w462, w460, "_T_1_C_L.txt" ("Suffix (transfer)")) -> (w513:string)
        n55 = VISA Write(VISA resource name=w483, write buffer=":PAGE:CHAN:MODE SWE;" ("write buffer (\"\")"), error in (no error)=w482) -> (VISA resource name out=w480:refnum<visa-resource-name>, error out=w481:errorcluster)  [unwired: 1 out]
        n56 = local read "Plot transfer curve extrema vs time"() -> (w410:bool)
        n57 = String To Path(string=w513) -> (path=w511:path)
        n58 = Index Array(array=w487, index #1=0 ("Index")) -> (element #1=w500:dbl, element #2=w499:dbl, element #3=w498:dbl)  [unwired: 2 in]
        n59 = Delete From Array(array=w487, length=3 ("Length"), index=0 ("Index")) -> (array with subset deleted=w485:dbl[])  [unwired: 1 out]
        n60 = case shown="True" w410 {
          tunnel: w459 -> [w516 w519]
          tunnel: w456 -> [_ w518]
          tunnel: [w516 w517] -> w428
          frame False {
          }
          frame True {
            n61 = Build Array (concatenate)(w519, w518) -> (w517:i32[])
          }
        }
        n62 = Bundle By Name(cluster=w492, "Gate Start"=w500, "Gate Stop"=w499, "Gate Step (linear only)"=w498, "Gate Compliance"=w509, "Range mode"=w476, "Range"=w475) -> (w477:T6)
        n63 = Index Array(array=w485, index #1=0 ("Index")) -> (element #1=w495:dbl, element #2=w494:dbl, element #3=w493:dbl)  [unwired: 2 in]
        n64 = call <vilib>:"compatOverwrite.vi"("overwrite (F)"=TRUE) -> ("overwrite?"=w466:T8)
        n65 = Bundle By Name(cluster=w491, "Drain Start"=w495, "Drain Stop"=w494, "Drain Step"=w493, "Drain Compliance"=w510, "Range mode"=w474, "Range"=w473) -> (w478:T7)
        n66 = call "4155C Transfer.vi"("VISA resource name in"=w480, "Gate"=w477, "Drain"=w478, "Timings"=w508, "error in (no error)"=w481, "SMU4"=w409, "sweep mode"=w501, "Panel Controls"=w468) -> ("VG"=w465:dbl[], "Outparams"=w472:T9, "VISA Resource Name out"=w507:refnum<visa-resource-name>, "IS"=w438:dbl[], "ID"=w439:dbl[], "IG"=w437:dbl[], "error out"=w457:errorcluster, "SMU4"=w469:dbl[])  [unwired: 12 in]
        n67 = Unbundle By Name(w472) -> ("V2 Step"=w471:dbl, "V2 Start"=w470:dbl, "Number of points"=w426:i32)
        n68 = call "4155C Split array.vi"("Number of VAR2 steps"=w426, "Y2 data in"=w439, "X data in"=w465, "Y1 data in"=w438, "Y3 data in"=w437, "error in (no error)"=w457) -> ("Array of clusters"=w458:cluster{"Y data in":dbl[], "X data in":dbl[]}[], "error out"=w414:errorcluster)  [unwired: 1 in]
        n69 = case shown="True" "Plot transfer curve extrema vs time" {
          tunnel: w464 -> [w528 w598]
          tunnel: w455 -> [w529 w593]
          tunnel: w441 -> [w522 w589]
          tunnel: w440 -> [w523 w588]
          tunnel: w439 -> [_ w585]
          tunnel: w438 -> [_ w583]
          tunnel: w437 -> [_ w582]
          tunnel: w436 -> [w530 w578]
          tunnel: w435 -> [w531 w577]
          tunnel: w434 -> [w526 w574]
          tunnel: w433 -> [w527 w573]
          tunnel: w432 -> [w521 w570]
          tunnel: w431 -> [w520 w569]
          tunnel: w430 -> [w525 w566]
          tunnel: w429 -> [w524 w565]
          tunnel: w428 -> [_ w558]
          tunnel: [w526 w553] -> w427
          tunnel: w426 -> [_ w552]
          tunnel: [w527 w551] -> w425
          tunnel: [w528 w550] -> w424
          tunnel: [w529 w549] -> w423
          tunnel: [w530 w548] -> w422
          tunnel: [w531 w547] -> w421
          tunnel: [w525 w546] -> w420
          tunnel: [w524 w545] -> w419
          tunnel: [w523 w544] -> w418
          tunnel: [w522 w543] -> w417
          tunnel: [w521 w542] -> w416
          tunnel: [w520 w541] -> w415
          tunnel: w414 -> [w532 w540]
          tunnel: [w532 w536] -> w413
          frame False {
          }
          frame True {
            # "Adjusts graph colors."
            # "Adjusts graph colors."
            # "Ion will be the middle element of the array. The calculation of the index is done only once, since Is, Id, and Ig have the same dimensions."
            # "abs(Ig)"
            # "abs(Is)"
            # "Y1: Is\nY2: Id\nY3: Ig"
            # "abs(Id)"
            # "Adjusts graph colors."
            # "Adjusts graph colors."
            # "Adjusts graph colors."
            n70 = Absolute Value(x=w583) -> (abs(x)=w568:dbl[])
            n71 = Absolute Value(x=w585) -> (abs(x)=w584:dbl[])
            n72 = Absolute Value(x=w582) -> (abs(x)=w571:dbl[])
            n73 = Array Size(array=w584) -> (size(s)=w592:i32)
            n74 = Divide(x=w592, y=2) -> (x/y=w535:dbl)
            n75 = Subtract(x=w535, y=1) -> (x-y=w534:dbl)
            n76 = Array Max & Min(array=w568) -> (max value=w575:dbl, min value=w576:dbl)  [unwired: 2 out]
            n77 = Array Max & Min(array=w584) -> (max value=w597:dbl, min value=w581:dbl)  [unwired: 2 out]
            n78 = Array Max & Min(array=w571) -> (max value=w580:dbl, min value=w579:dbl)  [unwired: 2 out]
            n79 = Index Array(array=w568, index=w534) -> (element=w559:dbl)
            n80 = Index Array(array=w568, index=0) -> (element=w560:dbl)
            n81 = Index Array(array=w584, index=w534) -> (element=w561:dbl)
            n82 = Index Array(array=w584, index=0) -> (element=w562:dbl)
            n83 = Index Array(array=w571, index=w534) -> (element=w564:dbl)
            n84 = Index Array(array=w571, index=0) -> (element=w563:dbl)
            n85 = local write "Ig max"(w580) -> ()
            n86 = local write "Ig min"(w579) -> ()
            n87 = local write "Is max"(w575) -> ()
            n88 = local write "Is min"(w576) -> ()
            n89 = local write "Id max"(w597) -> ()
            n90 = local write "Id min"(w581) -> ()
            n91 = Build Array (concatenate)(w574, w575) -> (w553:dbl[])
            n92 = Build Array (concatenate)(w573, w576) -> (w551:dbl[])
            n93 = local write "Is off"(w560) -> ()
            n94 = local write "Is on"(w559) -> ()
            n95 = Build Array (concatenate)(w598, w597) -> (w550:dbl[])
            n96 = Build Array (concatenate)(w593, w581) -> (w549:dbl[])
            n97 = Build Array (concatenate)(w578, w580) -> (w548:dbl[])
            n98 = Build Array (concatenate)(w577, w579) -> (w547:dbl[])
            n99 = Build Array (concatenate)(w566, w559) -> (w546:dbl[])
            n100 = Build Array (concatenate)(w565, w560) -> (w545:dbl[])
            n101 = Build Array (concatenate)(w588, w561) -> (w544:dbl[])
            n102 = Build Array (concatenate)(w589, w562) -> (w543:dbl[])
            n103 = Build Array (concatenate)(w570, w564) -> (w542:dbl[])
            n104 = Build Array (concatenate)(w569, w563) -> (w541:dbl[])
            n105 = local write "Ig off"(w563) -> ()
            n106 = local write "Ig on"(w564) -> ()
            n107 = local write "Id off"(w562) -> ()
            n108 = local write "Id on"(w561) -> ()
            n109 = control-ref of="Imax vs time"() -> (w587:refnum<vi>)
            n110 = control-ref of="Imin vs time"() -> (w586:refnum<vi>)
            n111 = control-ref of="Ion vs time"() -> (w555:refnum<vi>)
            n112 = control-ref of="Ioff vs time"() -> (w554:refnum<vi>)
            n113 = control-ref of="I vs Vg"() -> (w596:refnum<vi>)
            n114 = call "4155C Split array.vi"("Number of VAR2 steps"=w552, "Y2 data in"=w544, "X data in"=w558, "Y1 data in"=w546, "Y3 data in"=w542, "error in (no error)"=w540) -> ("Array of clusters"=w556:cluster{"Y data in":dbl[], "X data in":dbl[]}[], "error out"=w539:errorcluster)  [unwired: 1 in]
            n115 = call "4155C Split array.vi"("Number of VAR2 steps"=w552, "Y2 data in"=w543, "X data in"=w558, "Y1 data in"=w545, "Y3 data in"=w541, "error in (no error)"=w539) -> ("Array of clusters"=w557:cluster{"Y data in":dbl[], "X data in":dbl[]}[], "error out"=w538:errorcluster)  [unwired: 1 in]
            n116 = call "4155C Split array.vi"("Number of VAR2 steps"=w552, "Y2 data in"=w550, "X data in"=w558, "Y1 data in"=w553, "Y3 data in"=w548, "error in (no error)"=w538) -> ("Array of clusters"=w595:cluster{"Y data in":dbl[], "X data in":dbl[]}[], "error out"=w537:errorcluster)  [unwired: 1 in]
            n117 = call "4155C Split array.vi"("Number of VAR2 steps"=w552, "Y2 data in"=w549, "X data in"=w558, "Y1 data in"=w551, "Y3 data in"=w547, "error in (no error)"=w537) -> ("Array of clusters"=w594:cluster{"Y data in":dbl[], "X data in":dbl[]}[], "error out"=w536:errorcluster)  [unwired: 1 in]
            n118 = call "4155C Config Chart Colours.vi"("Numeric"=w552, "XY Graph 2"=w587) -> ()  [unwired: 6 in]
            n119 = call "4155C Config Chart Colours.vi"("Numeric"=w552, "XY Graph 2"=w586) -> ()  [unwired: 6 in]
            n120 = call "4155C Config Chart Colours.vi"("Numeric"=w552, "XY Graph 2"=w555) -> ()  [unwired: 6 in]
            n121 = call "4155C Config Chart Colours.vi"("Numeric"=w552, "XY Graph 2"=w554) -> ()  [unwired: 6 in]
            n122 = call "4155C Config Chart Colours.vi"("Numeric"=w552, "XY Graph 2"=w596) -> ()  [unwired: 6 in]
            n123 = local write "Imax vs time"(w595) -> ()
            n124 = local write "Imin vs time"(w594) -> ()
            n125 = local write "Ion vs time"(w556) -> ()
            n126 = local write "Ioff vs time"(w557) -> ()
          }
        }
        n127 = local write "I vs Vg"(w458) -> ()
        n128 = Open/Create/Replace File(file path (use dialog)=w511, error in=w413, operation (0:open)=w466) -> (refnum out=w453:refnum<file>, error out=w451:errorcluster)  [unwired: 3 in, 1 out]
        n129 = call "4155C Make Big 2d array.vi"("1D Var1"=w465, "1d IS"=w438, "1d ID"=w439, "1d IG"=w437, "1d SMU4"=w469, "SMU4"=w409, "VAR2 START"=w470, "Number of VAR2 steps"=w426, "VAR2 STEP"=w471, "VAR1 Name"="Vg", "Decimal places in header"=i8 1, "VAR2 Name"="Vd") -> ("Header array"=w454:string[], "Data array"=w452:dbl[][])  [unwired: 14 in]
        n130 = call "4155C Write array to file.vi"("Byte Stream File Refnum"=w453, "Header"=w454, "Data Array"=w452, "error in (no error)"=w451) -> ("dup refnum"=w450:refnum<file>, "error out"=w449:errorcluster)  [unwired: 1 in]
        n131 = Close File(refnum=w450, error in=w449) -> (error out=w506:errorcluster)  [unwired: 1 out]
      }
      frame "pulsedstressV" {
        w632 = 0
        n132 = Number To Decimal String(number=w623) -> (decimal integer string=w678:string)  [unwired: 1 in]
        n133 = Delete From Array(array=w613, index=0 ("Index")) -> (deleted portion=w669:string, array with subset deleted=w668:string[])  [unwired: 1 in]
        n134 = Bundle By Name(cluster=w649, "Emergency Stop"=w681) -> (w650:T2)
        n135 = VISA Write(VISA resource name=w662, write buffer=":PAGE:CHAN:MODE SWE;" ("write buffer (\"\")"), error in (no error)=w661) -> (VISA resource name out=w659:refnum<visa-resource-name>, error out=w660:errorcluster)  [unwired: 1 out]
        n136 = Concatenate Strings(w677, "-pulsedstressV-" ("Substring"), w678, w622, ".txt" ("Substring")) -> (w680:string)
        n137 = case shown="\"d\", Default" w669 {
          tunnel: [w690 w691] -> w667
          frame "s" {
            w690 = u16 0 items=["Single", "Double"] ("sweep mode")
          }
          frame "d", Default {
            w691 = u16 1 items=["Single", "Double"] ("sweep mode")
          }
        }
        n138 = Fract/Exp String To Number(string=w668) -> (number=w663:dbl[])  [unwired: 3 in, 1 out]
        n139 = String To Path(string=w680) -> (path=w676:path)
        n140 = Index Array(array=w663, index #1=0 ("Index")) -> (element #1=w641:dbl, element #2=w640:dbl, element #3=w637:dbl, element #4=w636:dbl, element #5=w635:dbl, element #6=w639:dbl)  [unwired: 5 in]
        n141 = Bundle By Name(cluster=w638, "Pulse period"=w636, "Base voltage"=w637, "Pulse width"=w635) -> (w634:T5)
        n142 = Unbundle By Name(w634) -> ("Pulse period"=w642:dbl)
        n143 = Bundle By Name(cluster=w665, "Gate Start"=w640, "Gate Stop"=w641, "Gate Step (linear only)"=0, "Gate Compliance"=w674, "Range mode"=w655, "Range"=w654) -> (w656:T6)
        n144 = call <vilib>:"compatOverwrite.vi"("overwrite (F)"=TRUE) -> ("overwrite?"=w627:T8)
        n145 = Bundle By Name(cluster=w664, "Drain Start"=w639, "Drain Stop"=w632, "Drain Step"=w632, "Drain Compliance"=w675, "Range mode"=w653, "Range"=w652) -> (w657:T7)
        n146 = call "4155C PulsedStressV.vi"("VISA resource name in"=w659, "sweep mode"=w667, "Panel Controls"=w650, "Gate"=w656, "Drain"=w657, "Timings"=w634, "error in (no error)"=w660, "SMU4"=w601) -> ("VISA Resource Name out"=w672:refnum<visa-resource-name>, "ID"=w630:dbl[], "IG"=w628:dbl[], "Outparams"=w651:T9, "error out"=w673:errorcluster)  [unwired: 3 in]
        n147 = Unbundle By Name(w651) -> ("Number of points"=w629:i32)  [unwired: 2 out]
        n148 = for {
          N: w629 -> [_]
          tunnel: [w687] -> w631 mode=indexing
          tunnel: w642 -> [w689]
          i -> [w688]
          n149 = Multiply(x=w689, y=w688) -> (x*y=w687:dbl)
        }
        n150 = Insert Into Array(array=dbl[][] [] ("Input Array"), new element=w631) -> (w643:dbl[][])  [unwired: 2 in]
        n151 = Insert Into Array(array=w643, new element=w630) -> (w648:dbl[][])  [unwired: 2 in]
        n152 = Insert Into Array(array=w648, new element=w628) -> (w647:dbl[][])  [unwired: 2 in]
        n153 = Transpose 2D Array(2D array=w647) -> (transposed array=w646:dbl[][])
        n154 = Open/Create/Replace File(file path (use dialog)=w676, error in=w673, operation (0:open)=w627) -> (refnum out=w684:refnum<file>, error out=w685:errorcluster)  [unwired: 3 in, 1 out]
        n155 = call "4155C Write array to file.vi"("Byte Stream File Refnum"=w684, "Header"=string[] ["Time /s", "Id /A", "Ig /A"], "Data Array"=w646, "error in (no error)"=w685) -> ("dup refnum"=w682:refnum<file>, "error out"=w683:errorcluster)  [unwired: 1 in]
        n156 = Close File(refnum=w682, error in=w683) -> (error out=w671:errorcluster)  [unwired: 1 out]
      }
      frame "transfer-fpp" {
        n157 = Number To Decimal String(number=w714) -> (decimal integer string=w768:string)  [unwired: 1 in]
        n158 = Bundle By Name(cluster=w744, "Emergency Stop"=w772) -> (w780:T1)
        n159 = Delete From Array(array=w759, index=0 ("Index")) -> (deleted portion=w757:string, array with subset deleted=w756:string[])  [unwired: 1 in]
        n160 = Concatenate Strings(w767, "-transferfpp-" ("Substring"), w768, w712, ".txt" ("Substring")) -> (w770:string)
        n161 = VISA Write(VISA resource name=w736, write buffer=":PAGE:CHAN:MODE SWE;" ("write buffer (\"\")"), error in (no error)=w735) -> (VISA resource name out=w733:refnum<visa-resource-name>, error out=w734:errorcluster)  [unwired: 1 out]
        n162 = case shown="\"d\", Default" w757 {
          tunnel: [w781 w782] -> w755
          frame "s" {
            w781 = u16 0 items=["Single", "Double"] ("sweep mode")
          }
          frame "d", Default {
            w782 = u16 1 items=["Single", "Double"] ("sweep mode")
          }
        }
        n163 = Fract/Exp String To Number(string=w756) -> (number=w740:dbl[])  [unwired: 3 in, 1 out]
        n164 = String To Path(string=w770) -> (path=w766:path)
        n165 = Index Array(array=w740, index #1=0 ("Index")) -> (element #1=w754:dbl, element #2=w753:dbl, element #3=w752:dbl)  [unwired: 2 in]
        n166 = Delete From Array(array=w740, length=3 ("Length"), index=0 ("Index")) -> (array with subset deleted=w738:dbl[])  [unwired: 1 out]
        n167 = Bundle By Name(cluster=w746, "Gate Start"=w754, "Gate Stop"=w753, "Gate Step (linear only)"=w752, "Gate Compliance"=w764, "Range mode"=w729, "Range"=w728) -> (w730:T6)
        n168 = Index Array(array=w738, index #1=0 ("Index")) -> (element #1=w749:dbl, element #2=w748:dbl, element #3=w747:dbl)  [unwired: 2 in]
        n169 = call <vilib>:"compatOverwrite.vi"("overwrite (F)"=TRUE) -> ("overwrite?"=w717:T8)
        n170 = Bundle By Name(cluster=w745, "Drain Start"=w749, "Drain Stop"=w748, "Drain Step"=w747, "Drain Compliance"=w765, "Range mode"=w727, "Range"=w726) -> (w731:T7)
        n171 = call "4155C Transfer-FPP.vi"("VISA resource name in"=w733, "Gate"=w730, "Drain"=w731, "Timings"=w763, "error in (no error)"=w734, "sweep mode"=w755, "Panel Controls"=w780) -> ("VG"=w771:dbl[], "Outparams"=w725:T9, "VISA Resource Name out"=w761:refnum<visa-resource-name>, "Vprobe2"=w721:dbl[], "ID"=w720:dbl[], "IG"=w719:dbl[], "Vprobe1"=w718:dbl[], "error out"=w762:errorcluster)  [unwired: 13 in]
        n172 = Unbundle By Name(w725) -> ("V2 Step"=w724:dbl, "V2 Start"=w723:dbl, "Number of points"=w722:i32)
        n173 = Open/Create/Replace File(file path (use dialog)=w766, error in=w762, operation (0:open)=w717) -> (refnum out=w777:refnum<file>, error out=w778:errorcluster)  [unwired: 3 in, 1 out]
        n174 = call "4155C Make Big 2d array FPP.vi"("1D Var1"=w771, "1d ID"=w720, "1d Vp2"=w721, "1d IG"=w719, "1d Vp1"=w718, "VAR2 START"=w723, "Number of VAR2 steps"=w722, "VAR2 STEP"=w724, "VAR1 Name"="Vg", "Decimal places in header"=i8 1, "VAR2 Name"="Vd") -> ("Header array"=w773:string[], "Data array"=w774:dbl[][])  [unwired: 15 in]
        n175 = call "4155C Write array to file.vi"("Byte Stream File Refnum"=w777, "Header"=w773, "Data Array"=w774, "error in (no error)"=w778) -> ("dup refnum"=w775:refnum<file>, "error out"=w776:errorcluster)  [unwired: 1 in]
        n176 = Close File(refnum=w775, error in=w776) -> (error out=w760:errorcluster)  [unwired: 1 out]
      }
      frame "output" {
        # "Is off"
        # "Is on"
        # "Ig off"
        # "Ig on"
        # "Is min"
        # "Is max"
        # "Ig min"
        # "Ig max"
        # "Id min"
        # "Id max"
        # "Id off"
        # "Id on"
        n177 = Delete From Array(array=w879, index=0 ("Index")) -> (deleted portion=w877:string, array with subset deleted=w876:string[])  [unwired: 1 in]
        n178 = Bundle By Name(cluster=w786, "Emergency Stop"=w888) -> (w842:T1)
        n179 = Number To Decimal String(number=w838) -> (decimal integer string=w837:string)  [unwired: 1 in]
        n180 = case shown="\"d\", Default" w877 {
          tunnel: [w973 w974] -> w875
          frame "s" {
            w973 = u16 0 items=["Single", "Double"] ("sweep mode")
          }
          frame "d", Default {
            w974 = u16 1 items=["Single", "Double"] ("sweep mode")
          }
        }
        n181 = Fract/Exp String To Number(string=w876) -> (number=w861:dbl[])  [unwired: 3 in, 1 out]
        n182 = Concatenate Strings(w886, w787, w837, w835, "_O_1_C_L.txt" ("Suffix (transfer)")) -> (w887:string)
        n183 = VISA Write(VISA resource name=w857, write buffer=":PAGE:CHAN:MODE SWE;" ("write buffer (\"\")"), error in (no error)=w856) -> (VISA resource name out=w854:refnum<visa-resource-name>, error out=w855:errorcluster)  [unwired: 1 out]
        n184 = String To Path(string=w887) -> (path=w885:path)
        n185 = local read "Plot output curve extrema vs time"() -> (w784:bool)
        n186 = Index Array(array=w861, index #1=0 ("Index")) -> (element #1=w874:dbl, element #2=w873:dbl, element #3=w872:dbl)  [unwired: 2 in]
        n187 = Delete From Array(array=w861, length=3 ("Length"), index=0 ("Index")) -> (array with subset deleted=w859:dbl[])  [unwired: 1 out]
        n188 = case shown="True" w784 {
          tunnel: w834 -> [w890 w893]
          tunnel: w831 -> [_ w892]
          tunnel: [w890 w891] -> w803
          frame False {
          }
          frame True {
            n189 = Build Array (concatenate)(w893, w892) -> (w891:i32[])
          }
        }
        n190 = Bundle By Name(cluster=w866, "Gate Start"=w874, "Gate Stop"=w873, "Gate Step (linear only)"=w872, "Gate Compliance"=w883, "Range mode"=w850, "Range"=w849) -> (w851:T6)
        n191 = Index Array(array=w859, index #1=0 ("Index")) -> (element #1=w869:dbl, element #2=w868:dbl, element #3=w867:dbl)  [unwired: 2 in]
        n192 = call <vilib>:"compatOverwrite.vi"("overwrite (F)"=TRUE) -> ("overwrite?"=w841:T8)
        n193 = Bundle By Name(cluster=w865, "Drain Start"=w869, "Drain Stop"=w868, "Drain Step"=w867, "Drain Compliance"=w884, "Range mode"=w848, "Range"=w847) -> (w852:T7)
        n194 = call "4155C Output.vi"("VISA resource name in"=w854, "Gate"=w851, "Drain"=w852, "Timings"=w882, "error in (no error)"=w855, "SMU4"=w783, "sweep mode"=w875, "Panel controls"=w842) -> ("VD"=w840:dbl[], "Outparams"=w846:T9, "VISA Resource Name out"=w881:refnum<visa-resource-name>, "IS"=w813:dbl[], "ID"=w814:dbl[], "IG"=w812:dbl[], "error out"=w832:errorcluster, "SMU4"=w843:dbl[])  [unwired: 12 in]
        n195 = Unbundle By Name(w846) -> ("V2 Step"=w845:dbl, "V2 Start"=w844:dbl, "Number of points"=w801:i32)
        n196 = call "4155C Split array.vi"("Number of VAR2 steps"=w801, "Y2 data in"=w814, "X data in"=w840, "Y1 data in"=w813, "Y3 data in"=w812, "error in (no error)"=w832) -> ("Array of clusters"=w833:cluster{"Y data in":dbl[], "X data in":dbl[]}[], "error out"=w789:errorcluster)  [unwired: 1 in]
        n197 = case shown="True" "Plot output curve extrema vs time" {
          tunnel: w839 -> [w897 w972]
          tunnel: w830 -> [w896 w967]
          tunnel: w816 -> [w902 w963]
          tunnel: w815 -> [w903 w962]
          tunnel: w814 -> [_ w959]
          tunnel: w813 -> [_ w957]
          tunnel: w812 -> [_ w956]
          tunnel: w811 -> [w895 w952]
          tunnel: w810 -> [w894 w951]
          tunnel: w809 -> [w899 w948]
          tunnel: w808 -> [w898 w947]
          tunnel: w807 -> [w901 w944]
          tunnel: w806 -> [w900 w943]
          tunnel: w805 -> [w905 w940]
          tunnel: w804 -> [w904 w939]
          tunnel: w803 -> [_ w932]
          tunnel: [w899 w927] -> w802
          tunnel: w801 -> [_ w926]
          tunnel: [w898 w925] -> w800
          tunnel: [w897 w924] -> w799
          tunnel: [w896 w923] -> w798
          tunnel: [w895 w922] -> w797
          tunnel: [w894 w921] -> w796
          tunnel: [w905 w920] -> w795
          tunnel: [w904 w919] -> w794
          tunnel: [w903 w918] -> w793
          tunnel: [w902 w917] -> w792
          tunnel: [w901 w916] -> w791
          tunnel: [w900 w915] -> w790
          tunnel: w789 -> [w906 w914]
          tunnel: [w906 w910] -> w788
          frame False {
          }
          frame True {
            # "Adjusts graph colors."
            # "Adjusts graph colors."
            # "Ion will be the middle element of the array. The calculation of the index is done only once, since Is, Id, and Ig have the same dimensions."
            # "abs(Ig)"
            # "abs(Is)"
            # "Y1: Is\nY2: Id\nY3: Ig"
            # "abs(Id)"
            # "Adjusts graph colors."
            # "Adjusts graph colors."
            # "Adjusts graph colors."
            n198 = Absolute Value(x=w957) -> (abs(x)=w942:dbl[])
            n199 = Absolute Value(x=w959) -> (abs(x)=w958:dbl[])
            n200 = Absolute Value(x=w956) -> (abs(x)=w945:dbl[])
            n201 = Array Size(array=w958) -> (size(s)=w966:i32)
            n202 = Divide(x=w966, y=2) -> (x/y=w909:dbl)
            n203 = Subtract(x=w909, y=1) -> (x-y=w908:dbl)
            n204 = Array Max & Min(array=w942) -> (max value=w949:dbl, min value=w950:dbl)  [unwired: 2 out]
            n205 = Array Max & Min(array=w958) -> (max value=w971:dbl, min value=w955:dbl)  [unwired: 2 out]
            n206 = Array Max & Min(array=w945) -> (max value=w954:dbl, min value=w953:dbl)  [unwired: 2 out]
            n207 = Index Array(array=w942, index=w908) -> (element=w933:dbl)
            n208 = Index Array(array=w942, index=0) -> (element=w934:dbl)
            n209 = Index Array(array=w958, index=w908) -> (element=w935:dbl)
            n210 = Index Array(array=w958, index=0) -> (element=w936:dbl)
            n211 = Index Array(array=w945, index=w908) -> (element=w938:dbl)
            n212 = Index Array(array=w945, index=0) -> (element=w937:dbl)
            n213 = local write "Ig max"(w954) -> ()
            n214 = local write "Ig min"(w953) -> ()
            n215 = local write "Is max"(w949) -> ()
            n216 = local write "Is min"(w950) -> ()
            n217 = local write "Id max"(w971) -> ()
            n218 = local write "Id min"(w955) -> ()
            n219 = Build Array (concatenate)(w948, w949) -> (w927:dbl[])
            n220 = Build Array (concatenate)(w947, w950) -> (w925:dbl[])
            n221 = local write "Is off"(w934) -> ()
            n222 = local write "Is on"(w933) -> ()
            n223 = Build Array (concatenate)(w972, w971) -> (w924:dbl[])
            n224 = Build Array (concatenate)(w967, w955) -> (w923:dbl[])
            n225 = Build Array (concatenate)(w952, w954) -> (w922:dbl[])
            n226 = Build Array (concatenate)(w951, w953) -> (w921:dbl[])
            n227 = Build Array (concatenate)(w940, w933) -> (w920:dbl[])
            n228 = Build Array (concatenate)(w939, w934) -> (w919:dbl[])
            n229 = Build Array (concatenate)(w962, w935) -> (w918:dbl[])
            n230 = Build Array (concatenate)(w963, w936) -> (w917:dbl[])
            n231 = Build Array (concatenate)(w944, w938) -> (w916:dbl[])
            n232 = Build Array (concatenate)(w943, w937) -> (w915:dbl[])
            n233 = local write "Ig off"(w937) -> ()
            n234 = local write "Ig on"(w938) -> ()
            n235 = local write "Id off"(w936) -> ()
            n236 = local write "Id on"(w935) -> ()
            n237 = control-ref of="Imax vs time"() -> (w961:refnum<vi>)
            n238 = control-ref of="Imin vs time"() -> (w960:refnum<vi>)
            n239 = control-ref of="Ion vs time"() -> (w929:refnum<vi>)
            n240 = control-ref of="Ioff vs time"() -> (w928:refnum<vi>)
            n241 = control-ref of="I vs Vg"() -> (w970:refnum<vi>)
            n242 = call "4155C Split array.vi"("Number of VAR2 steps"=w926, "Y2 data in"=w918, "X data in"=w932, "Y1 data in"=w920, "Y3 data in"=w916, "error in (no error)"=w914) -> ("Array of clusters"=w930:cluster{"Y data in":dbl[], "X data in":dbl[]}[], "error out"=w913:errorcluster)  [unwired: 1 in]
            n243 = call "4155C Split array.vi"("Number of VAR2 steps"=w926, "Y2 data in"=w917, "X data in"=w932, "Y1 data in"=w919, "Y3 data in"=w915, "error in (no error)"=w913) -> ("Array of clusters"=w931:cluster{"Y data in":dbl[], "X data in":dbl[]}[], "error out"=w912:errorcluster)  [unwired: 1 in]
            n244 = call "4155C Split array.vi"("Number of VAR2 steps"=w926, "Y2 data in"=w924, "X data in"=w932, "Y1 data in"=w927, "Y3 data in"=w922, "error in (no error)"=w912) -> ("Array of clusters"=w969:cluster{"Y data in":dbl[], "X data in":dbl[]}[], "error out"=w911:errorcluster)  [unwired: 1 in]
            n245 = call "4155C Split array.vi"("Number of VAR2 steps"=w926, "Y2 data in"=w923, "X data in"=w932, "Y1 data in"=w925, "Y3 data in"=w921, "error in (no error)"=w911) -> ("Array of clusters"=w968:cluster{"Y data in":dbl[], "X data in":dbl[]}[], "error out"=w910:errorcluster)  [unwired: 1 in]
            n246 = call "4155C Config Chart Colours.vi"("Numeric"=w926, "XY Graph 2"=w961) -> ()  [unwired: 6 in]
            n247 = call "4155C Config Chart Colours.vi"("Numeric"=w926, "XY Graph 2"=w960) -> ()  [unwired: 6 in]
            n248 = call "4155C Config Chart Colours.vi"("Numeric"=w926, "XY Graph 2"=w929) -> ()  [unwired: 6 in]
            n249 = call "4155C Config Chart Colours.vi"("Numeric"=w926, "XY Graph 2"=w928) -> ()  [unwired: 6 in]
            n250 = call "4155C Config Chart Colours.vi"("Numeric"=w926, "XY Graph 2"=w970) -> ()  [unwired: 6 in]
            n251 = local write "Imax vs time"(w969) -> ()
            n252 = local write "Imin vs time"(w968) -> ()
            n253 = local write "Ion vs time"(w930) -> ()
            n254 = local write "Ioff vs time"(w931) -> ()
          }
        }
        n255 = local write "I vs Vd"(w833) -> ()
        n256 = Open/Create/Replace File(file path (use dialog)=w885, error in=w788, operation (0:open)=w841) -> (refnum out=w828:refnum<file>, error out=w826:errorcluster)  [unwired: 3 in, 1 out]
        n257 = call "4155C Make Big 2d array.vi"("1D Var1"=w840, "1d IS"=w813, "1d ID"=w814, "1d IG"=w812, "1d SMU4"=w843, "SMU4"=w783, "VAR2 START"=w844, "Number of VAR2 steps"=w801, "VAR2 STEP"=w845, "VAR1 Name"="Vd", "Decimal places in header"=i8 1, "VAR2 Name"="Vg") -> ("Header array"=w829:string[], "Data array"=w827:dbl[][])  [unwired: 14 in]
        n258 = call "4155C Write array to file.vi"("Byte Stream File Refnum"=w828, "Header"=w829, "Data Array"=w827, "error in (no error)"=w826) -> ("dup refnum"=w825:refnum<file>, "error out"=w824:errorcluster)  [unwired: 1 in]
        n259 = Close File(refnum=w825, error in=w824) -> (error out=w880:errorcluster)  [unwired: 1 out]
      }
      frame "output-fpp" {
        n260 = Number To Decimal String(number=w996) -> (decimal integer string=w1050:string)  [unwired: 1 in]
        n261 = Bundle By Name(cluster=w1026, "Emergency Stop"=w1053) -> (w1063:T1)
        n262 = Delete From Array(array=w1041, index=0 ("Index")) -> (deleted portion=w1039:string, array with subset deleted=w1038:string[])  [unwired: 1 in]
        n263 = VISA Write(VISA resource name=w1017, write buffer=":PAGE:CHAN:MODE SWE;" ("write buffer (\"\")"), error in (no error)=w1014) -> (VISA resource name out=w1016:refnum<visa-resource-name>, error out=w1015:errorcluster)  [unwired: 1 out]
        n264 = Concatenate Strings(w1049, "-outputfpp-" ("Substring"), w1050, w995, ".txt" ("Substring")) -> (w1052:string)
        n265 = case shown="\"d\", Default" w1039 {
          tunnel: [w1064 w1065] -> w1037
          frame "s" {
            w1064 = u16 0 items=["Single", "Double"] ("sweep mode")
          }
          frame "d", Default {
            w1065 = u16 1 items=["Single", "Double"] ("sweep mode")
          }
        }
        n266 = Fract/Exp String To Number(string=w1038) -> (number=w1020:dbl[])  [unwired: 3 in, 1 out]
        n267 = String To Path(string=w1052) -> (path=w1048:path)
        n268 = Index Array(array=w1020, index #1=0 ("Index")) -> (element #1=w1036:dbl, element #2=w1035:dbl, element #3=w1034:dbl)  [unwired: 2 in]
        n269 = Delete From Array(array=w1020, length=3 ("Length"), index=0 ("Index")) -> (array with subset deleted=w1019:dbl[])  [unwired: 1 out]
        n270 = Bundle By Name(cluster=w1028, "Gate Start"=w1036, "Gate Stop"=w1035, "Gate Step (linear only)"=w1034, "Gate Compliance"=w1046, "Range mode"=w1012, "Range"=w1011) -> (w1062:T6)
        n271 = Index Array(array=w1019, index #1=0 ("Index")) -> (element #1=w1031:dbl, element #2=w1030:dbl, element #3=w1029:dbl)  [unwired: 2 in]
        n272 = call <vilib>:"compatOverwrite.vi"("overwrite (F)"=TRUE) -> ("overwrite?"=w1000:T8)
        n273 = Bundle By Name(cluster=w1027, "Drain Start"=w1031, "Drain Stop"=w1030, "Drain Step"=w1029, "Drain Compliance"=w1047, "Range mode"=w1010, "Range"=w1013) -> (w1061:T7)
        n274 = call "4155C Output-FPP.vi"("VISA resource name in"=w1016, "Gate"=w1062, "Drain"=w1061, "Timings"=w1045, "error in (no error)"=w1015, "sweep mode"=w1037, "Panel controls"=w1063) -> ("VD"=w1005:dbl[], "Outparams"=w1008:T9, "VISA Resource Name out"=w1043:refnum<visa-resource-name>, "Vprobe2"=w1004:dbl[], "ID"=w1003:dbl[], "IG"=w1002:dbl[], "Vprobe1"=w1001:dbl[], "error out"=w1044:errorcluster)  [unwired: 13 in]
        n275 = Unbundle By Name(w1008) -> ("V2 Step"=w1009:dbl, "V2 Start"=w1007:dbl, "Number of points"=w1006:i32)
        n276 = Open/Create/Replace File(file path (use dialog)=w1048, error in=w1044, operation (0:open)=w1000) -> (refnum out=w1058:refnum<file>, error out=w1059:errorcluster)  [unwired: 3 in, 1 out]
        n277 = call "4155C Make Big 2d array FPP.vi"("1D Var1"=w1005, "1d ID"=w1003, "1d Vp2"=w1004, "1d IG"=w1002, "1d Vp1"=w1001, "VAR2 START"=w1007, "Number of VAR2 steps"=w1006, "VAR2 STEP"=w1009, "VAR1 Name"="Vd", "Decimal places in header"=i8 1, "VAR2 Name"="Vg") -> ("Header array"=w1054:string[], "Data array"=w1055:dbl[][])  [unwired: 15 in]
        n278 = call "4155C Write array to file.vi"("Byte Stream File Refnum"=w1058, "Header"=w1054, "Data Array"=w1055, "error in (no error)"=w1059) -> ("dup refnum"=w1056:refnum<file>, "error out"=w1057:errorcluster)  [unwired: 1 in]
        n279 = Close File(refnum=w1056, error in=w1057) -> (error out=w1042:errorcluster)  [unwired: 1 out]
      }
      frame "itime" {
        n280 = Delete From Array(array=w1069, index=1) -> (deleted portion=w1068:string)  [unwired: 1 in, 1 out]
        n281 = Delete From Array(array=w1069, index=0 ("Index")) -> (deleted portion=w1103:string)  [unwired: 1 in, 1 out]
        n282 = Fract/Exp String To Number(string=w1068) -> (number=w1067:dbl)  [unwired: 3 in, 1 out]
        n283 = case shown="\"l\"" w1103 {
          tunnel: w1102 -> [w1108 w1110 w1114]
          tunnel: [w1107 w1109 w1113] -> w1095
          tunnel: w1067 -> [w1105 _ w1112]
          frame "s" {
            w1106 = u32 0 items=["short  ", "medium  ", "long  "] ("integration time 2")
            n284 = Bundle By Name(cluster=w1108, "integration time"=w1106, "Short/Long integration time"=w1105) -> (w1107:T5)
          }
          frame "m", Default {
            w1111 = u32 1 items=["short  ", "medium  ", "long  "] ("integration time 2")
            n285 = Bundle By Name(cluster=w1110, "integration time"=w1111) -> (w1109:T5)
          }
          frame "l" {
            w1115 = u32 2 items=["short  ", "medium  ", "long  "] ("integration time 2")
            n286 = Bundle By Name(cluster=w1114, "integration time"=w1115, "Short/Long integration time"=w1112) -> (w1113:T5)
          }
        }
      }
      frame "pulsed" {
        n287 = Delete From Array(array=w1150, index=0 ("Index")) -> (deleted portion=w1151:string, array with subset deleted=w1138:string[])  [unwired: 1 in]
        n288 = case shown="\"on\", Default" w1151 {
          tunnel: w1149 -> [w1161 w1164]
          tunnel: [w1160 w1163] -> w1142
          tunnel: w1138 -> [w1158 _]
          frame "on", Default {
            w1159 = u16 1 items=["Continuous", "Pulsed"] ("sweep method")
            n289 = Fract/Exp String To Number(string=w1158) -> (number=w1156:dbl[])  [unwired: 3 in, 1 out]
            n290 = Index Array(array=w1156, index #1=0 ("Index")) -> (element #1=w1155:dbl, element #2=w1154:dbl, element #3=w1153:dbl)  [unwired: 2 in]
            n291 = Bundle By Name(cluster=w1161, "sweep method"=w1159, "Pulse period"=w1155, "Base voltage"=w1154, "Pulse width"=w1153) -> (w1160:T5)
          }
          frame "off" {
            w1162 = u16 0 items=["Continuous", "Pulsed"] ("sweep method")
            n292 = Bundle By Name(cluster=w1164, "sweep method"=w1162) -> (w1163:T5)
          }
        }
      }
      frame "gaterangemode" {
        n293 = Delete From Array(array=w1197, index=0 ("Index")) -> (deleted portion=w1198:string)  [unwired: 1 in, 1 out]
        n294 = case shown="\"f\"" w1198 {
          tunnel: [w1200 w1201 w1202] -> w1187
          frame "a", Default {
            w1200 = u16 0 items=["Auto", "Limited", "Fixed"] ("Gate Range\nmode 2")
          }
          frame "f" {
            w1201 = u16 2 items=["Auto", "Limited", "Fixed"] ("Gate Range\nmode 2")
          }
          frame "l" {
            w1202 = u16 1 items=["Auto", "Limited", "Fixed"] ("Gate Range\nmode 2")
          }
        }
      }
      frame "gaterange" {
        (unwired) u8 11 items=["10fA  ", "100fA  ", "1nA  ", "10nA", "100nA", "1uA", "10uA", "100uA", "1mA", "10mA", "100mA", "1A"] ("Gate Range 2")
        n295 = Delete From Array(array=w1242, index=0 ("Index")) -> (deleted portion=w1232:string)  [unwired: 1 in, 1 out]
        n296 = Scan Value(string=w1232, format string="") -> (value=w1230:dbl)  [unwired: 1 in, 1 out]
        n297 = Logarithm Base 10(1:w1230) -> (0:w1229:dbl)
        n298 = Round To Nearest(number=w1229) -> (nearest integer value=w1228:dbl)
        n299 = Add(x=w1228, y=11.0) -> (x+y=w1226:dbl)
        n300 = To Unsigned Byte Integer(number=w1226) -> (unsigned 8bit integer=w1225:u8)
      }
      frame "drainrange" {
        (unwired) u8 11 items=["10fA  ", "100fA  ", "1nA  ", "10nA", "100nA", "1uA", "10uA", "100uA", "1mA", "10mA", "100mA", "1A"] ("Gate Range 2")
        n301 = Delete From Array(array=w1283, index=0 ("Index")) -> (deleted portion=w1274:string)  [unwired: 1 in, 1 out]
        n302 = Scan Value(string=w1274, format string="") -> (value=w1272:dbl)  [unwired: 1 in, 1 out]
        n303 = Logarithm Base 10(1:w1272) -> (0:w1271:dbl)
        n304 = Round To Nearest(number=w1271) -> (nearest integer value=w1270:dbl)
        n305 = Add(x=w1270, y=11.0) -> (x+y=w1268:dbl)
        n306 = To Unsigned Byte Integer(number=w1268) -> (unsigned 8bit integer=w1267:u8)
      }
      frame "drainrangemode" {
        n307 = Delete From Array(array=w1317, index=0 ("Index")) -> (deleted portion=w1318:string)  [unwired: 1 in, 1 out]
        n308 = case shown="\"f\"" w1318 {
          tunnel: [w1320 w1321 w1322] -> w1307
          frame "a", Default {
            w1320 = u16 0 items=["Auto", "Limited", "Fixed"] ("Gate Range\nmode 2")
          }
          frame "f" {
            w1321 = u16 2 items=["Auto", "Limited", "Fixed"] ("Gate Range\nmode 2")
          }
          frame "l" {
            w1322 = u16 1 items=["Auto", "Limited", "Fixed"] ("Gate Range\nmode 2")
          }
        }
      }
      frame "Error", Default {
      }
      frame "logfile" {
        n309 = Number To Decimal String(number=w1377) -> (decimal integer string=w1412:string)  [unwired: 1 in]
        n310 = Concatenate Strings(w1411, "logfile" ("Substring"), w1412, w1375, ".txt" ("Substring")) -> (w1409:string)
        n311 = String To Path(string=w1409) -> (path=w1382:path)
        n312 = Unbundle(w1408) -> ("integration time"=w1407:u32, "Short/Long integration time"=w1406:dbl, "hold time (sec)"=w1405:dbl, "delay time (sec)"=w1404:dbl, "Step Time (0 disables)"=w1403:dbl, "sweep method"=w1402:u16, "Pulse period"=w1401:dbl, "Base voltage"=w1400:dbl, "Pulse width"=w1399:dbl)
        n313 = Build Array(w1407, w1406, w1405, w1404, w1403, w1402, w1401, w1400, w1399, w1393, w1394, w1395, w1396, w1397, w1398) -> (w1386:dbl[])
        n314 = Insert Into Array(array=dbl[][] [] ("Input Array"), new element=w1386) -> (w1385:dbl[][])  [unwired: 2 in]
        n315 = call <vilib>:"compatOverwrite.vi"("overwrite (F)"=TRUE) -> ("overwrite?"=w1380:T8)
        n316 = Open/Create/Replace File(file path (use dialog)=w1382, error in=w1384, operation (0:open)=w1380) -> (refnum out=w1390:refnum<file>, error out=w1389:errorcluster)  [unwired: 3 in, 1 out]
        n317 = call "4155C Write array to file.vi"("Byte Stream File Refnum"=w1390, "Header"=string[] ["Int Time", "Short/Long Itime", "Hold time", "Delay time", "Step time", "Sweep method", "Pulse period", "Base Voltage", "Pulse width", "Drain compliance", "Gate compliance", "Gate range mode", "Gate range", "S/D range mode", "S/D range"], "Data Array"=w1385, "error in (no error)"=w1389) -> ("dup refnum"=w1392:refnum<file>, "error out"=w1391:errorcluster)  [unwired: 1 in]
        n318 = Close File(refnum=w1392, error in=w1391) -> (error out=w1383:errorcluster)  [unwired: 1 out]
      }
      frame "sample" {
        n319 = Number To Decimal String(number=w1436) -> (decimal integer string=w1484:string)  [unwired: 1 in]
        n320 = Fract/Exp String To Number(string=w1481) -> (number=w1442:dbl[])  [unwired: 3 in, 1 out]
        n321 = Concatenate Strings(w1459, "-sample-" ("Substring"), w1484, w1434, ".txt" ("Substring")) -> (w1482:string)
        n322 = Index Array(array=w1442, index=0 ("Index")) -> (element=w1479:dbl)
        n323 = String To Path(string=w1482) -> (path=w1463:path)
        n324 = Index Array(array=w1442, index=2 ("Index")) -> (element=w1475:dbl)
        n325 = Index Array(array=w1442, index=3 ("Index")) -> (element=w1444:dbl)
        n326 = Index Array(array=w1442, index=4 ("Index")) -> (element=w1441:dbl)
        n327 = call "4155C Config Sampling Measurements.vi"("Sampling interval"=w1441, "Sample time"=w1444, "Display on/off"=TRUE, "Timings"=w1450, "Num Points"=w1475, "error in (no error)"=w1486, "Drain Compliance"=w1485, "Gate Compliance"=w1460, "VISA session"=w1487) -> ("error out"=w1488:errorcluster, "dup VISA resource name"=w1489:refnum<visa-resource-name>)  [unwired: 1 in]
        n328 = Index Array(array=w1442, index=1 ("Index")) -> (element=w1476:dbl)
        n329 = call "4155C Take Sample.vi"("Emergency Stop"=w1456, "error in (no error)"=w1488, "Vd"=w1476, "Vg"=w1479, "VISA resource name in"=w1489) -> ("error out"=w1454:errorcluster, "Id"=w1491:dbl[], "Ig"=w1465:dbl[], "VISA Resource Name out"=w1452:refnum<visa-resource-name>, "Is"=w1490:dbl[], "Time"=w1469:dbl[])  [unwired: 1 in]
        n330 = Insert Into Array(array=dbl[][] [] ("Input Array"), new element=w1469) -> (w1468:dbl[][])  [unwired: 2 in]
        n331 = Insert Into Array(array=w1468, new element=w1465) -> (w1467:dbl[][])  [unwired: 2 in]
        n332 = Insert Into Array(array=w1467, new element=w1491) -> (w1466:dbl[][])  [unwired: 2 in]
        n333 = VISA Write(VISA resource name=w1452, write buffer=":DISP ON" ("write buffer (\"\")"), error in (no error)=w1454) -> (VISA resource name out=w1451:refnum<visa-resource-name>, error out=w1453:errorcluster)  [unwired: 1 out]
        n334 = Insert Into Array(array=w1466, new element=w1490) -> (w1458:dbl[][])  [unwired: 2 in]
        n335 = Transpose 2D Array(2D array=w1458) -> (transposed array=w1457:dbl[][])
        n336 = call <vilib>:"compatOverwrite.vi"("overwrite (F)"=TRUE) -> ("overwrite?"=w1439:T8)
        n337 = Open/Create/Replace File(file path (use dialog)=w1463, error in=w1453, operation (0:open)=w1439) -> (refnum out=w1472:refnum<file>, error out=w1471:errorcluster)  [unwired: 3 in, 1 out]
        n338 = call "4155C Write array to file.vi"("Byte Stream File Refnum"=w1472, "Header"=string[] ["Time /s", "Ig /A", "Id /A", "Is /A"], "Data Array"=w1457, "error in (no error)"=w1471) -> ("dup refnum"=w1474:refnum<file>, "error out"=w1473:errorcluster)  [unwired: 1 in]
        n339 = Close File(refnum=w1474, error in=w1473) -> (error out=w1461:errorcluster)  [unwired: 1 out]
      }
      frame "samplei" {
        n340 = Number To Decimal String(number=w1514) -> (decimal integer string=w1565:string)  [unwired: 1 in]
        n341 = Concatenate Strings(w1544, "-samplei-" ("Substring"), w1565, w1513, ".txt" ("Substring")) -> (w1563:string)
        n342 = Fract/Exp String To Number(string=w1562) -> (number=w1529:dbl[])  [unwired: 3 in, 1 out]
        n343 = String To Path(string=w1563) -> (path=w1547:path)
        n344 = Index Array(array=w1529, index=4 ("Index")) -> (element=w1523:dbl)
        n345 = Index Array(array=w1529, index=3 ("Index")) -> (element=w1524:dbl)
        n346 = Index Array(array=w1529, index=1 ("Index")) -> (element=w1526:dbl)
        n347 = Index Array(array=w1529, index=0 ("Index")) -> (element=w1527:dbl)
        n348 = Index Array(array=w1529, index=2 ("Index")) -> (element=w1525:dbl)
        n349 = call "4155C Config SamplingI Measurements.vi"("Sample time"=w1525, "Display on/off"=TRUE, "Timings"=w1536, "Num Points"=w1526, "error in (no error)"=w1567, "Sampling interval"=w1524, "VISA session"=w1568) -> ("error out"=w1569:errorcluster, "dup VISA resource name"=w1570:refnum<visa-resource-name>)  [unwired: 3 in]
        n350 = call "4155C Take SampleI.vi"("Emergency Stop"=w1541, "error in (no error)"=w1569, "Idg 2"=w1527, "Vdg compliance 2"=w1523, "VISA resource name in"=w1570) -> ("error out"=w1539:errorcluster, "Idg"=w1572:dbl[], "Vdg"=w1549:dbl[], "VISA Resource Name out"=w1537:refnum<visa-resource-name>, "Is"=w1571:dbl[], "Time"=w1553:dbl[])  [unwired: 1 in]
        n351 = Insert Into Array(array=dbl[][] [] ("Input Array"), new element=w1553) -> (w1552:dbl[][])  [unwired: 2 in]
        n352 = Insert Into Array(array=w1552, new element=w1549) -> (w1551:dbl[][])  [unwired: 2 in]
        n353 = Insert Into Array(array=w1551, new element=w1572) -> (w1550:dbl[][])  [unwired: 2 in]
        n354 = VISA Write(VISA resource name=w1537, write buffer=":DISP ON" ("write buffer (\"\")"), error in (no error)=w1539) -> (VISA resource name out=w1522:refnum<visa-resource-name>, error out=w1538:errorcluster)  [unwired: 1 out]
        n355 = Insert Into Array(array=w1550, new element=w1571) -> (w1543:dbl[][])  [unwired: 2 in]
        n356 = call <vilib>:"compatOverwrite.vi"("overwrite (F)"=TRUE) -> ("overwrite?"=w1517:T8)
        n357 = Open/Create/Replace File(file path (use dialog)=w1547, error in=w1538, operation (0:open)=w1517) -> (refnum out=w1556:refnum<file>, error out=w1555:errorcluster)  [unwired: 3 in, 1 out]
        n358 = Transpose 2D Array(2D array=w1543) -> (transposed array=w1542:dbl[][])
        n359 = call "4155C Write array to file.vi"("Byte Stream File Refnum"=w1556, "Header"=string[] ["Time /s", "Vdg /V", "Idg /A", "Is /A"], "Data Array"=w1542, "error in (no error)"=w1555) -> ("dup refnum"=w1558:refnum<file>, "error out"=w1557:errorcluster)  [unwired: 1 in]
        n360 = Close File(refnum=w1558, error in=w1557) -> (error out=w1520:errorcluster)  [unwired: 1 out]
        n361 = VISA Write(VISA resource name=w1522, write buffer=";:PAGE:SCON:STAN OFF;:PAGE:CHAN:VSU2:DIS;" ("write buffer (\"\")"), error in (no error)=w1520) -> (VISA resource name out=w1518:refnum<visa-resource-name>, error out=w1519:errorcluster)  [unwired: 1 out]
      }
      frame "#" {
        n362 = VISA Write(VISA resource name=w1599, write buffer=":DISP ON" ("write buffer (\"\")"), error in (no error)=w1598) -> (VISA resource name out=w1597:refnum<visa-resource-name>, error out=w1596:errorcluster)  [unwired: 1 out]
      }
      frame "stressV" {
        n363 = Number To Decimal String(number=w1629) -> (decimal integer string=w1670:string)  [unwired: 1 in]
        n364 = Concatenate Strings(w1654, "-stressV-" ("Substring"), w1670, w1628, ".txt" ("Substring")) -> (w1668:string)
        n365 = Fract/Exp String To Number(string=w1667) -> (number=w1640:dbl[])  [unwired: 3 in, 1 out]
        n366 = String To Path(string=w1668) -> (path=w1658:path)
        n367 = Index Array(array=w1640, index=3 ("Index")) -> (element=w1637:dbl)
        n368 = Index Array(array=w1640, index=1 ("Index")) -> (element=w1635:dbl)
        n369 = Index Array(array=w1640, index=0 ("Index")) -> (element=w1634:dbl)
        n370 = Index Array(array=w1640, index=4 ("Index")) -> (element=w1639:dbl)
        n371 = Index Array(array=w1640, index=2 ("Index")) -> (element=w1636:dbl)
        n372 = call "4155C Config V Stress.vi"("VISA session"=w1673, "ID compliance"=w1637, "VD"=w1635, "VG"=w1634, "IG compliance"=w1636, "error in (no error)"=w1672, "Display on/off"=TRUE) -> ("dup VISA resource name"=w1675:refnum<visa-resource-name>, "error out"=w1674:errorcluster)
        n373 = call "4155C Apply Stress.vi"("error in (no error)"=w1674, "Duration"=w1639, "Emergency Stop"=w1653, "VISA resource name in"=w1675) -> ("error out"=w1651:errorcluster, "VISA Resource Name out"=w1649:refnum<visa-resource-name>)
        n374 = VISA Write(VISA resource name=w1649, write buffer=":DISP ON" ("write buffer (\"\")"), error in (no error)=w1651) -> (VISA resource name out=w1648:refnum<visa-resource-name>, error out=w1650:errorcluster)  [unwired: 1 out]
        n375 = call <vilib>:"compatOverwrite.vi"("overwrite (F)"=TRUE) -> ("overwrite?"=w1633:T8)
        n376 = Open/Create/Replace File(file path (use dialog)=w1658, error in=w1650, operation (0:open)=w1633) -> (refnum out=w1661:refnum<file>, error out=w1660:errorcluster)  [unwired: 3 in, 1 out]
        n377 = call "4155C Write array to file.vi"("Byte Stream File Refnum"=w1661, "Header"=string[] ["V stress completed successfully", ""], "error in (no error)"=w1660) -> ("dup refnum"=w1663:refnum<file>, "error out"=w1662:errorcluster)  [unwired: 2 in]
        n378 = Close File(refnum=w1663, error in=w1662) -> (error out=w1656:errorcluster)  [unwired: 1 out]
      }
      frame "stressI" {
        n379 = Number To Decimal String(number=w1697) -> (decimal integer string=w1734:string)  [unwired: 1 in]
        n380 = Concatenate Strings(w1718, "-stressI-" ("Substring"), w1734, w1696, ".txt" ("Substring")) -> (w1732:string)
        n381 = Fract/Exp String To Number(string=w1731) -> (number=w1706:dbl[])  [unwired: 3 in, 1 out]
        n382 = Index Array(array=w1706, index=1 ("Index")) -> (element=w1702:dbl)
        n383 = Index Array(array=w1706, index=0 ("Index")) -> (element=w1703:dbl)
        n384 = call "4155C Config I Stress.vi"("VISA session"=w1737, "IDG"=w1703, "VDG compliance"=w1702, "error in (no error)"=w1736, "Display on/off"=TRUE) -> ("dup VISA resource name"=w1739:refnum<visa-resource-name>, "error out"=w1738:errorcluster)
        n385 = Index Array(array=w1706, index=2 ("Index")) -> (element=w1704:dbl)
        n386 = String To Path(string=w1732) -> (path=w1722:path)
        n387 = call "4155C Apply Stress.vi"("error in (no error)"=w1738, "Duration"=w1704, "Emergency Stop"=w1717, "VISA resource name in"=w1739) -> ("error out"=w1715:errorcluster, "VISA Resource Name out"=w1713:refnum<visa-resource-name>)
        n388 = VISA Write(VISA resource name=w1713, write buffer=":DISP ON" ("write buffer (\"\")"), error in (no error)=w1715) -> (VISA resource name out=w1712:refnum<visa-resource-name>, error out=w1714:errorcluster)  [unwired: 1 out]
        n389 = call <vilib>:"compatOverwrite.vi"("overwrite (F)"=TRUE) -> ("overwrite?"=w1701:T8)
        n390 = Open/Create/Replace File(file path (use dialog)=w1722, error in=w1714, operation (0:open)=w1701) -> (refnum out=w1725:refnum<file>, error out=w1724:errorcluster)  [unwired: 3 in, 1 out]
        n391 = call "4155C Write array to file.vi"("Byte Stream File Refnum"=w1725, "Header"=string[] ["I stress completed successfully", ""], "error in (no error)"=w1724) -> ("dup refnum"=w1727:refnum<file>, "error out"=w1726:errorcluster)  [unwired: 2 in]
        n392 = Close File(refnum=w1727, error in=w1726) -> (error out=w1720:errorcluster)  [unwired: 1 out]
      }
      frame "vsu2pulse" {
        n393 = Number To Decimal String(number=w1761) -> (decimal integer string=w1796:string)  [unwired: 1 in]
        n394 = Concatenate Strings(w1781, "-vsu2-" ("Substring"), w1796, w1760, ".txt" ("Substring")) -> (w1794:string)
        n395 = Fract/Exp String To Number(string=w1793) -> (number=w1769:dbl[])  [unwired: 3 in, 1 out]
        n396 = String To Path(string=w1794) -> (path=w1785:path)
        n397 = Index Array(array=w1769, index=1 ("Index")) -> (element=w1768:dbl)
        n398 = Index Array(array=w1769, index=0 ("Index")) -> (element=w1766:dbl)
        n399 = call "4155C Config VSU2 Stress.vi"("error in (no error)"=w1798, "VSU2"=w1766, "Display on/off"=TRUE, "VISA session"=w1799) -> ("error out"=w1800:errorcluster, "dup VISA resource name"=w1801:refnum<visa-resource-name>)
        n400 = call "4155C Apply Stress.vi"("error in (no error)"=w1800, "Duration"=w1768, "Emergency Stop"=w1780, "VISA resource name in"=w1801) -> ("error out"=w1778:errorcluster, "VISA Resource Name out"=w1776:refnum<visa-resource-name>)
        n401 = VISA Write(VISA resource name=w1776, write buffer=":DISP ON" ("write buffer (\"\")"), error in (no error)=w1778) -> (VISA resource name out=w1775:refnum<visa-resource-name>, error out=w1777:errorcluster)  [unwired: 1 out]
        n402 = call <vilib>:"compatOverwrite.vi"("overwrite (F)"=TRUE) -> ("overwrite?"=w1765:T8)
        n403 = Open/Create/Replace File(file path (use dialog)=w1785, error in=w1777, operation (0:open)=w1765) -> (refnum out=w1788:refnum<file>, error out=w1787:errorcluster)  [unwired: 3 in, 1 out]
        n404 = call "4155C Write array to file.vi"("Byte Stream File Refnum"=w1788, "Header"=string[] ["VSU2 pulse completed successfully", ""], "error in (no error)"=w1787) -> ("dup refnum"=w1790:refnum<file>, "error out"=w1789:errorcluster)  [unwired: 2 in]
        n405 = Close File(refnum=w1790, error in=w1789) -> (error out=w1783:errorcluster)  [unwired: 1 out]
      }
      frame "sample-fpp" {
        w1834 = string[] ["Time /s", "Id VgVd /A", "Ig VgVd /A", "Vp1 VgVd /V", "Vp2 VgVd /V"] ("Header")
        w1838 = "%d" ("format string")
        n406 = Number To Decimal String(number=w1823) -> (decimal integer string=w1886:string)  [unwired: 1 in]
        n407 = Fract/Exp String To Number(string=w1883) -> (number=w1871:dbl[])  [unwired: 3 in, 1 out]
        n408 = Concatenate Strings(w1877, "-samplefpp-" ("Substring"), w1886, w1822, ".txt" ("Substring")) -> (w1884:string)
        n409 = String To Path(string=w1884) -> (path=w1846:path)
        n410 = Index Array(array=w1871, index=0 ("Index")) -> (element=w1832:dbl)
        n411 = Index Array(array=w1871, index=1 ("Index")) -> (element=w1831:dbl)
        n412 = Index Array(array=w1871, index=2 ("Index")) -> (element=w1879:dbl)
        n413 = Index Array(array=w1871, index=3 ("Index")) -> (element=w1869:dbl)
        n414 = call "4155C Config Sampling Measurements FPP.vi"("VISA session"=w1889, "Num Points"=w1879, "Vg"=w1832, "Display on/off"=TRUE, "Gate Compliance"=w1878, "Drain Compliance"=w1887, "Standby"="Standby", "error in (no error)"=w1888, "Timings"=w1876, "Vd"=w1831, "Sample time"=w1869) -> ("dup VISA resource name"=w1848:refnum<visa-resource-name>, "error out"=w1847:errorcluster)  [unwired: 3 in]
        n415 = Number To Decimal String(number=w1832) -> (decimal integer string=w1858:string)  [unwired: 1 in]
        n416 = call "4155C Take Sample FPP.vi"("VISA resource name in"=w1848, "error in (no error)"=w1847, "Emergency Stop"=w1849) -> ("Time"=w1853:dbl[], "Vp1"=w1863:dbl[], "VISA Resource Name out"=w1829:refnum<visa-resource-name>, "Ig"=w1851:dbl[], "Id"=w1852:dbl[], "Vp2"=w1861:dbl[], "error out"=w1850:errorcluster)  [unwired: 10 in]
        n417 = Insert Into Array(array=dbl[][] [] ("Input Array"), new element=w1853) -> (w1867:dbl[][])  [unwired: 2 in]
        n418 = Number To Decimal String(number=w1831) -> (decimal integer string=w1856:string)  [unwired: 1 in]
        n419 = Insert Into Array(array=w1867, new element=w1852) -> (w1866:dbl[][])  [unwired: 2 in]
        n420 = Concatenate Strings("(Vg = " ("Substring"), w1858, "V, Vd = " ("Substring"), w1856, "V)" ("Substring")) -> (w1854:string)
        n421 = Insert Into Array(array=w1866, new element=w1851) -> (w1865:dbl[][])  [unwired: 2 in]
        n422 = Insert Into Array(array=w1865, new element=w1863) -> (w1862:dbl[][])  [unwired: 2 in]
        n423 = Insert Into Array(array=w1862, new element=w1861) -> (w1830:dbl[][])  [unwired: 2 in]
        n424 = Transpose 2D Array(2D array=w1830) -> (transposed array=w1860:dbl[][])
        n425 = call <vilib>:"compatOverwrite.vi"("overwrite (F)"=TRUE) -> ("overwrite?"=w1827:T8)
        n426 = Open/Create/Replace File(file path (use dialog)=w1846, error in=w1850, operation (0:open)=w1827) -> (refnum out=w1843:refnum<file>, error out=w1844:errorcluster)  [unwired: 3 in, 1 out]
        n427 = Array To Spreadsheet String(array=w1834, 3:w1838) -> (spreadsheet string=w1840:string)  [unwired: 1 in]
        n428 = Search and Replace String(replace all?=TRUE ("replace all? (F)"), input string=w1840, search string="VgVd", replace string=w1854) -> (result string=w1836:string)  [unwired: 4 in, 3 out]
        n429 = Spreadsheet String To Array(format string=w1838, spreadsheet string=w1836, array type (2D Dbl)=w1834) -> (array=w1835:string[])  [unwired: 1 in]
        n430 = call "4155C Write array to file.vi"("Byte Stream File Refnum"=w1843, "Header"=w1835, "Data Array"=w1860, "error in (no error)"=w1844) -> ("dup refnum"=w1841:refnum<file>, "error out"=w1842:errorcluster)  [unwired: 1 in]
        n431 = Close File(refnum=w1841, error in=w1842) -> (error out=w1828:errorcluster)  [unwired: 1 out]
      }
      frame "resample-fpp" {
        w1924 = string[] ["Time /s", "Id VgVd /A", "Ig VgVd /A", "Vp1 VgVd /V", "Vp2 VgVd /V"] ("Header")
        w1928 = "%d" ("format string")
        n432 = Number To Decimal String(number=w1910) -> (decimal integer string=w1968:string)  [unwired: 1 in]
        n433 = Fract/Exp String To Number(string=w1965) -> (number=w1917:dbl[])  [unwired: 3 in, 1 out]
        n434 = Concatenate Strings(w1961, "-resamplefpp-" ("Substring"), w1968, w1911, ".txt" ("Substring")) -> (w1966:string)
        n435 = String To Path(string=w1966) -> (path=w1936:path)
        n436 = Index Array(array=w1917, index=0 ("Index")) -> (element=w1923:dbl)
        n437 = Index Array(array=w1917, index=1 ("Index")) -> (element=w1922:dbl)
        n438 = Number To Decimal String(number=w1923) -> (decimal integer string=w1946:string)  [unwired: 1 in]
        n439 = call "4155C Take Sample FPP.vi"("VISA resource name in"=w1919, "error in (no error)"=w1918, "Emergency Stop"=w1937) -> ("Time"=w1941:dbl[], "Vp1"=w1951:dbl[], "VISA Resource Name out"=w1921:refnum<visa-resource-name>, "Ig"=w1939:dbl[], "Id"=w1940:dbl[], "Vp2"=w1949:dbl[], "error out"=w1938:errorcluster)  [unwired: 10 in]
        n440 = Insert Into Array(array=dbl[][] [] ("Input Array"), new element=w1941) -> (w1955:dbl[][])  [unwired: 2 in]
        n441 = Number To Decimal String(number=w1922) -> (decimal integer string=w1944:string)  [unwired: 1 in]
        n442 = Insert Into Array(array=w1955, new element=w1940) -> (w1954:dbl[][])  [unwired: 2 in]
        n443 = Concatenate Strings("(Vg = " ("Substring"), w1946, "V, Vd = " ("Substring"), w1944, "V)" ("Substring")) -> (w1942:string)
        n444 = Insert Into Array(array=w1954, new element=w1939) -> (w1953:dbl[][])  [unwired: 2 in]
        n445 = Insert Into Array(array=w1953, new element=w1951) -> (w1950:dbl[][])  [unwired: 2 in]
        n446 = Insert Into Array(array=w1950, new element=w1949) -> (w1916:dbl[][])  [unwired: 2 in]
        n447 = call <vilib>:"compatOverwrite.vi"("overwrite (F)"=TRUE) -> ("overwrite?"=w1915:T8)
        n448 = Open/Create/Replace File(file path (use dialog)=w1936, error in=w1938, operation (0:open)=w1915) -> (refnum out=w1933:refnum<file>, error out=w1934:errorcluster)  [unwired: 3 in, 1 out]
        n449 = Array To Spreadsheet String(array=w1924, 3:w1928) -> (spreadsheet string=w1930:string)  [unwired: 1 in]
        n450 = Transpose 2D Array(2D array=w1916) -> (transposed array=w1948:dbl[][])
        n451 = Search and Replace String(replace all?=TRUE ("replace all? (F)"), input string=w1930, search string="VgVd", replace string=w1942) -> (result string=w1926:string)  [unwired: 4 in, 3 out]
        n452 = Spreadsheet String To Array(format string=w1928, spreadsheet string=w1926, array type (2D Dbl)=w1924) -> (array=w1925:string[])  [unwired: 1 in]
        n453 = call "4155C Write array to file.vi"("Byte Stream File Refnum"=w1933, "Header"=w1925, "Data Array"=w1948, "error in (no error)"=w1934) -> ("dup refnum"=w1931:refnum<file>, "error out"=w1932:errorcluster)  [unwired: 1 in]
        n454 = Close File(refnum=w1931, error in=w1932) -> (error out=w1920:errorcluster)  [unwired: 1 out]
      }
      frame "serial" {
        n455 = local read "Termination char\n(0xA = '\\n' = LF)\n(0xD = '\\r' = CR)"() -> (w1997:u8)
        n456 = local read "Enable Termination\nChar (T)"() -> (w1998:bool)
        n457 = Index Array(array=w2005, index=0 ("Index")) -> (element=w2004:string)
        n458 = local read "parity"() -> (w1988:u16)
        n459 = local read "Delay before read (ms)"() -> (w1999:u32)
        n460 = local read "byte count"() -> (w1996:u32)
        n461 = local read "Timeout (ms)"() -> (w1995:u32)
        n462 = local read "VISA resource name"() -> (w1992:refnum<visa-resource-name>)
        n463 = local read "baud rate"() -> (w1991:u32)
        n464 = local read "Serial End Mode for Reads"() -> (w1990:u16)
        n465 = local read "data bits"() -> (w1989:u16)
        n466 = local read "stop bits"() -> (w1994:u16)
        n467 = local read "flow control"() -> (w1993:u16)
        n468 = call "Serial write and read v0.5.vi"("Delay before read (ms)"=w1999, "Termination char\n(0xA = '\\n' = LF)\n(0xD = '\\r' = CR)"=w1997, "Enable Termination\nChar (T)"=w1998, "parity"=w1988, "stop bits"=w1994, "string to write"=w2004, "flow control"=w1993, "byte count"=w1996, "Serial Settings:Serial End Mode for Reads"=w1990, "Timeout (ms)"=w1995, "error in (no error)"=w2010, "VISA resource name"=w1992, "baud rate"=w1991, "data bits"=w1989) -> ("Serial port output"=w2000:string, "error out"=w2009:errorcluster)
        n469 = Build Array (concatenate)(w2000, w2001) -> (w2002:string[])
      }
      frame "pump" {
        # "Time array for valve position"
        # "Time array for absolute plunger position"
        # "Valve position"
        # "Absolute plunger position"
        # "Remove \"_\""
        # "Check if hard stop is pressed."
        # "Check if halt is pressed."
        # "Check if pump is idle. Else halt."
        n470 = Index Array(array=w2076, index=0 ("Index")) -> (element=w2053:string)
        n471 = case shown="\"No error\", Default" w2051 {
          tunnel: w2053 -> [w2112 _ w2114 w2115 w2116 w2117 _ _ w2120 w2121 _]
          tunnel: [w2112 "/1H" w2114 w2115 w2116 w2117 "/1H" "/1H" w2120 w2121 "/1H"] -> w2052
          frame "No error", Default {
          }
          frame "Initialization" {
          }
          frame "Invalid command" {
          }
          frame "Invalid operand" {
          }
          frame "Device not initialized" {
          }
          frame "Internal failure" {
          }
          frame "Plunger overload" {
          }
          frame "Valve overload" {
          }
          frame "Plunger move not allowed" {
          }
          frame "A/D converter failure" {
          }
          frame "Command overflow" {
          }
        }
        n472 = local read "Hard stop pump"() -> (w2055:bool)
        n473 = local read "Halt pump"() -> (w2058:bool)
        n474 = local read "Serial End Mode for Reads"() -> (w2064:u16)
        n475 = local read "flow control"() -> (w2067:u16)
        n476 = local read "stop bits"() -> (w2068:u16)
        n477 = local read "parity"() -> (w2062:u16)
        n478 = local read "Delay before read (ms)"() -> (w2073:u32)
        n479 = local read "byte count"() -> (w2070:u32)
        n480 = local read "Timeout (ms)"() -> (w2069:u32)
        n481 = local read "VISA resource name"() -> (w2066:refnum<visa-resource-name>)
        n482 = local read "baud rate"() -> (w2065:u32)
        n483 = local read "Enable Termination\nChar (T)"() -> (w2072:bool)
        n484 = local read "Termination char\n(0xA = '\\n' = LF)\n(0xD = '\\r' = CR)"() -> (w2071:u8)
        n485 = case shown="True" w2058 {
          tunnel: [w2126 "/1H"] -> w2057
          tunnel: w2052 -> [w2126 _]
          frame False {
          }
          frame True {
            n486 = local write "Halt pump"(FALSE) -> ()
          }
        }
        n487 = case shown="True" w2055 {
          tunnel: [w2123 "/1T"] -> w2056
          tunnel: w2057 -> [w2123 _]
          frame False {
          }
          frame True {
            n488 = local write "Hard stop pump"(FALSE) -> ()
          }
        }
        n489 = local read "data bits"() -> (w2063:u16)
        n490 = String Subset(string=w2047, offset (0)=1) -> (substring=w2045:string)  [unwired: 1 in]
        n491 = call "SPM Pump v0.6.vi"("Termination char\n(0xA = '\\n' = LF)\n(0xD = '\\r' = CR)"=w2071, "Enable Termination\nChar (T)"=w2072, "Timeout (ms)"=w2069, "Serial Settings:Serial End Mode for Reads"=w2064, "byte count"=w2070, "Delay before read (ms)"=w2073, "Time <input>"=w2050, "error in (no error)"=w2081, "Serial port input"=w2056, "VISA resource name"=w2066, "parity"=w2062, "baud rate"=w2065, "stop bits"=w2068, "data bits"=w2063, "flow control"=w2067, "Time units <input>"=w2045) -> ("Input command"=w2044:string, "Serial port data"=w2034:string[], "Pump status"=w2040:string, "Valve position"=w2042:i32, "Absolute plunger position"=w2054:i32, "Serial port"=w2049:string, "error out"=w2080:errorcluster)  [unwired: 1 in, 4 out]
        n492 = case shown="\"?6\"" w2044 {
          tunnel: [w2093 w2101 w2107] -> w2061
          tunnel: w2060 -> [w2093 w2100 w2107]
          tunnel: w2054 -> [_ w2099 _]
          tunnel: w2041 -> [w2092 w2098 w2108]
          tunnel: [w2092 w2098 w2110] -> w2043
          tunnel: w2042 -> [_ _ w2109]
          tunnel: w2039 -> [_ w2097 w2105]
          tunnel: w2038 -> [w2091 w2096 w2106]
          tunnel: [w2091 w2095 w2106] -> w2037
          tunnel: [w2090 w2094 w2104] -> w2036
          tunnel: w2035 -> [w2090 w2094 w2103]
          frame "Q", Default {
          }
          frame "?" {
            n493 = Build Array (concatenate)(w2100, w2099) -> (w2101:i32[])
            n494 = Build Array (concatenate)(w2096, w2097) -> (w2095:i32[])
            n495 = call "4155C Split array.vi"("X data in"=w2095, "Y1 data in"=w2101) -> ("Array of clusters"=w2102:cluster{"Y data in":dbl[], "X data in":dbl[]}[])  [unwired: 5 in, 1 out]
            n496 = local write "Absolute plunger position vs time"(w2102) -> ()
          }
          frame "?6" {
            n497 = Build Array (concatenate)(w2108, w2109) -> (w2110:i32[])
            n498 = Build Array (concatenate)(w2103, w2105) -> (w2104:i32[])
            n499 = call "4155C Split array.vi"("X data in"=w2104, "Y1 data in"=w2110) -> ("Array of clusters"=w2111:cluster{"Y data in":dbl[], "X data in":dbl[]}[])  [unwired: 5 in, 1 out]
            n500 = local write "Valve position vs time"(w2111) -> ()
          }
        }
        n501 = Build Array (concatenate)(w2032, w2034) -> (w2033:string[][])
        n502 = Build Array (concatenate)(w2048, w2049) -> (w2074:string[])
      }
      frame "filename" {
        n503 = Index Array(array=w2131, index=0 ("Index")) -> (element=w2130:string)
      }
    }
    n504 = local read "Time Units"() -> (w71:u16)
    n505 = case shown="2" w71 {
      tunnel: ["Time (Seconds)" ("element") "Time (Minutes)" ("element") "Time (Hours)" ("element")] -> w111
      frame 0 {
      }
      frame 1, Default {
      }
      frame 2 {
      }
    }
    n506 = Build Array(w150, w79, w89, w88, w87, w86, w85, w84, w83, w82, w81, w80, w78) -> (w189:dbl[][])
    n507 = Transpose 2D Array(2D array=w189) -> (transposed array=w188:dbl[][])
    n508 = Concatenate Strings(w130, w73, "Imax_Imin_Ion_Ioff_vs_time.txt" ("Suffix (Imax,Imin,Ion,Ioff)")) -> (w199:string)
    n509 = Build Array(w111, "Is max (A)" ("VAR2 Name"), "Is min (A)" ("VAR2 Name"), "Id max (A)" ("VAR2 Name"), "Id min (A)" ("VAR2 Name"), "Ig max (A)" ("VAR2 Name"), "Ig min (A)" ("VAR2 Name"), "Is on (A)" ("VAR2 Name"), "Is off (A)" ("VAR2 Name"), "Id on (A)" ("VAR2 Name"), "Id off (A)" ("VAR2 Name"), "Ig on (A)" ("VAR2 Name"), "Ig off (A)" ("VAR2 Name")) -> (w194:string[])
    n510 = Array To Spreadsheet String(array=w188, 3:"%e" ("format string")) -> (spreadsheet string=w192:string)  [unwired: 1 in]
    n511 = Array To Spreadsheet String(array=w194, 3:"" ("format string")) -> (spreadsheet string=w193:string)  [unwired: 1 in]
    n512 = String To Path(string=w199) -> (path=w198:path)
    n513 = Build Array(w193, w192) -> (w191:string[])
    n514 = Write to Text File(file (use dialog)=w198, text=w191, error in=w146) -> (refnum out=w200:refnum<file>, error out=w190:errorcluster)  [unwired: 1 in, 1 out]
    n515 = Close File(refnum=w200, error in=w190) -> (error out=w129:errorcluster)  [unwired: 1 out]
    n516 = Build Array(w125, w151) -> (w156:i32[][])
    n517 = Build Array(w111, "Absolute plunger position" ("VAR2 Name")) -> (w159:string[])
    n518 = Transpose 2D Array(2D array=w156) -> (transposed array=w149:i32[][])
    n519 = Array To Spreadsheet String(array=w159, 3:"" ("format string")) -> (spreadsheet string=w158:string)  [unwired: 1 in]
    n520 = Array To Spreadsheet String(array=w149, 3:"%e" ("format string")) -> (spreadsheet string=w155:string)  [unwired: 1 in]
    n521 = Build Array(w158, w155) -> (w161:string[])
    n522 = Concatenate Strings(w130, w73, "plunger_vs_time.txt" ("Suffix (plunger)")) -> (w153:string)
    n523 = String To Path(string=w153) -> (path=w152:path)
    n524 = Write to Text File(file (use dialog)=w152, text=w161, error in=w129) -> (refnum out=w154:refnum<file>, error out=w163:errorcluster)  [unwired: 1 in, 1 out]
    n525 = Close File(refnum=w154, error in=w163) -> (error out=w128:errorcluster)  [unwired: 1 out]
    n526 = Concatenate Strings(w130, w73, "serial_port_output.txt" ("Suffix (serial port log)")) -> (w169:string)
    n527 = String To Path(string=w169) -> (path=w168:path)
    n528 = Build Array(w111, "Serial port input" ("VAR2 Name"), "Pump status" ("VAR2 Name"), "Serial port output: ") -> (w115:string[])
    n529 = Array To Spreadsheet String(array=w121, 3:"" ("format string")) -> (spreadsheet string=w112:string)  [unwired: 1 in]
    n530 = Array To Spreadsheet String(array=w115, 3:"" ("format string")) -> (spreadsheet string=w113:string)  [unwired: 1 in]
    n531 = Array To Spreadsheet String(array=w120, 3:"" ("format string")) -> (spreadsheet string=w174:string)  [unwired: 1 in]
    n532 = Build Array(w113, w112) -> (w114:string[])
    n533 = Write to Text File(file (use dialog)=w168, text=w114, error in=w128) -> (refnum out=w170:refnum<file>, error out=w171:errorcluster)  [unwired: 1 in, 1 out]
    n534 = local write "Serial port data"(w174) -> ()
    n535 = Close File(refnum=w170, error in=w171) -> (error out=w127:errorcluster)  [unwired: 1 out]
    n536 = Build Array(w124, w132) -> (w138:i32[][])
    n537 = Build Array(w111, "Valve port" ("VAR2 Name")) -> (w141:string[])
    n538 = Transpose 2D Array(2D array=w138) -> (transposed array=w133:i32[][])
    n539 = Array To Spreadsheet String(array=w141, 3:"" ("format string")) -> (spreadsheet string=w140:string)  [unwired: 1 in]
    n540 = Array To Spreadsheet String(array=w133, 3:"%e" ("format string")) -> (spreadsheet string=w137:string)  [unwired: 1 in]
    n541 = Build Array(w140, w137) -> (w143:string[])
    n542 = Concatenate Strings(w130, w73, "valve_port_vs_time.txt" ("Suffix (valve)")) -> (w135:string)
    n543 = String To Path(string=w135) -> (path=w134:path)
    n544 = Write to Text File(file (use dialog)=w134, text=w143, error in=w127) -> (refnum out=w136:refnum<file>, error out=w145:errorcluster)  [unwired: 1 in, 1 out]
    n545 = Close File(refnum=w136, error in=w145) -> (error out=w126:errorcluster)  [unwired: 1 out]
  }
  "error out" <- w32
  "Timings Indicator" <- w16
  "SMU4 Indicator" <- w1
  "Is max" <- w14
  "Id max" <- w14
  "Ig max" <- w14
  "Imax vs time" <- w10
  "I vs Vg" <- w10
  "Imin vs time" <- w10
  "I vs Vd" <- w10
  "Serial port data" <- "" ("Serial port data")
  "Valve position vs time" <- cluster{"Y data in":dbl[], "X data in":dbl[]}[] [] ("Valve position vs time")
  "Is min" <- w13
  "Id min" <- w13
  "Ig min" <- w13
  "Ion vs time" <- w10
  "Ioff vs time" <- w10
  "Is on" <- w12
  "Id on" <- w12
  "Ig on" <- w12
  "Is off" <- w11
  "Id off" <- w11
  "Ig off" <- w11
